vi "Example_Path to VCluster.vi"() -> ()   [LabVIEW 2015]
uses:
  <vilib>/addons/_JKI.lib/Serialization/JSON/JKI JSON Serialization.lvlib
panel:
  out "data":cluster{i32[][]}
  in  "input string":string="{\n\"History\": {\n    \"ZenParamsSpecVersion\": \"1.0.0\",\n    \"ModificationHistory\": [\n      {\n        \"DateModified\": \"19-07-2017\",\n        \"ModifiedBy\": \"SR\",\n        \"ModificationNotes\": \"FCI First version\",\n        \"DocumentVefrsion\": \"1.0.0\"\n      }\n    ],\n    \"ServiceHistory\": [\n      {\n        \"DateServiced\": \"23-03-2017\",\n        \"ServicedBy\": \"ABC\",\n        \"NextServiceDate\": \"23-03-2018\",\n        \"ServiceList\": {\n          \"CameraCalibrationDate\": \"2\",\n          \"CameraCalibrationFilePath\": \"C:\\\\Cam\",\n          \"SensorCalibration\": true,\n          \"SensorCalibNotes\": \"ReplacementDone\",\n          \"MotorCalib\": true,\n          \"MotorCalibNotes\": \"blah\"\n        },\n        \"ServiceNotes\": \"First version\"\n      },\n      {\n        \"DateServiced\": \"23-03-2017\",\n        \"ServicedBy\": \"ABC\",\n        \"NextServiceDate\": \"23-03-2018\",\n\"ServiceList\": {\n          \"CameraCalibrationDate\": \"2\",\n          \"CameraCalibrationFilePath\": \"C:\\\\Cam\",\n          \"SensorCalibration\": true,\n          \"SensorCalibNotes\": \"ReplacementDone\",\n          \"MotorCalib\": true,\n          \"MotorCalibNotes\": \"blah\"\n        },\n        \"ServiceNotes\": \"First version\"\n      }\n    ]\n  },\n  \"SystemParameters\": {\n    \"SystemName\": \"MolexGP2_001\",\n    \"SystemID\": \"GTRON1\",\n    \"CusftomerName\": \"Molex\",\n    \"Location\": \"Gandhinagar\",\n    \"InstallationfDate\": \"01-08-2015\",\n    \"NextServiceDate\": \"01-05-2017\",\n    \"CompatibleZenGageVersion\": \"2.0\",\n    \"NumberOfRacks\": 1,\n    \"TotalNumberOfCameras\": 3,\n    \"SoftwareFeatures\": {\n      \"ArduinoDiagnosticsEnableOnPowerOn\": true,\n      \"MotorDiagnosticsEnableOnPowerOn\": true,\n      \"CameraOpticsDiagnosticsEnableOnPowerOn\": false,\n      \"DefectTrackingEnable\": true,\n      \"AnalyticsEnable\": true,\n      \"DataLoggingEnable\": false,\n      \"ReportEnable\": false,\n      \"DeveloperMode\": false,\n      \"PauseOnReelCountFinish\": true,\n      \"PauseOnTotalCountFinish\": true,\n      \"DebugLevel\": 0,\n      \"SaveFailImages\": false\n    }\n  },\n  \"PartsConfigured\": [\n    {\n      \"Name\": \"102\",\n      \"NumberOfRack\": 1\n    }\n  ],\n  \"RackControllerParameters\": [\n    {\n      \"RackId\": 0,\n      \"PartsList\": [\n        {\n          \"Name\": \"102\",\n          \"ControlLimitsViolationThreshold\": {\n            \"M1\": 1,\n            \"N1\": 1\n          },\n          \"SpecificationLimitViolationThreshold\": {\n            \"M2\": 1,\n            \"N2\": 1\n          },\n          \"RejectPositionCount\": 106,\n          \"NumberOfCameras\": 1\n        },\n        {\n          \"Name\": \"122\",\n          \"ControlLimitsViolationThreshold\": {\n            \"M1\": 1,\n            \"N1\": 1\n          },\n          \"SpecificationLimitViolationThreshold\": {\n            \"M2\": 1,\n            \"N2\": 1\n          },\n          \"RejectPositionCount\": 77,\n          \"NumberOfCameras\": 3\n        },\n        {\n          \"Name\": \"145\",\n          \"ControlLimitsViolationThreshold\": {\n            \"M1\": 1,\n            \"N1\": 1\n          },\n          \"SpecificationLimitViolationThreshold\": {\n            \"M2\": 1,\n            \"N2\": 1\n          },\n          \"RejectPositionCount\": 78,\n          \"NumberOfCameras\": 3\n        },\n        {\n          \"Name\": \"162\",\n          \"ControlLimitsViolationThreshold\": {\n            \"M1\": 1,\n            \"N1\": 1\n          },\n          \"SpecificationLimitViolationThreshold\": {\n            \"M2\": 1,\n            \"N2\": 1\n          },\n          \"RejectPositionCount\": 78,\n          \"NumberOfCameras\": 3\n        },\n        {\n          \"Name\": \"182\",\n          \"ControlLimitsViolationThreshold\": {\n            \"M1\": 1,\n            \"N1\": 1\n          },\n          \"SpecificationLimitViolationThreshold\": {\n            \"M2\": 1,\n            \"N2\": 1\n          },\n          \"RejectPositionCount\": 78,\n          \"NumberOfCameras\": 3\n        },\n        {\n          \"Name\": \"175\",\n          \"ControlLimitsViolationThreshold\": {\n            \"M1\": 1,\n            \"N1\": 1\n          },\n          \"SpecificationLimitViolationThreshold\": {\n            \"M2\": 1,\n            \"N2\": 1\n          },\n          \"RejectPositionCount\": 78,\n          \"NumberOfCameras\": 3\n        },\n        {\n          \"Name\": \"130\",\n          \"ControlLimitsViolationThreshold\": {\n            \"M1\": 1,\n            \"N1\": 1\n          },\n          \"SpecificationLimitViolationThreshold\": {\n            \"M2\": 1,\n            \"N2\": 1\n          },\n          \"RejectPositionCount\": 78,\n          \"NumberOfCameras\": 3\n        },\n        {\n          \"Name\": \"142\",\n          \"ControlLimitsViolationThreshold\": {\n            \"M1\": 10,\n            \"N1\": 10\n          },\n          \"SpecificationLimitViolationThreshold\": {\n            \"M2\": 10,\n            \"N2\": 10\n          },\n          \"RejectPositionCount\": 78,\n          \"NumberOfCameras\": 3\n        },\n        {\n          \"Name\": \"160\",\n          \"ControlLimitsViolationThreshold\": {\n            \"M1\": 1,\n            \"N1\": 1\n          },\n          \"SpecificationLimitViolationThreshold\": {\n            \"M2\": 1,\n            \"N2\": 1\n          },\n          \"RejectPositionCount\": 78,\n          \"NumberOfCameras\": 3\n        }\n      ]\n    }\n  ],\n  \"CameraControllerParameters\": [\n    {\n      \"ID\": 0,\n      \"NoOfCameras\": 3,\n      \"CameraID\": [\n        0,\n        1,\n        2\n      ],\n      \"NoOfReceivers\": 1,\n      \"Diagnostics\": {\n        \"Path\": \"xxxxxx\",\n        \"LightCameraSequence\": [\n          {\n            \"Name\": \"LightCameraSequence1\",\n            \"CameraID\": 0,\n            \"LightID\": 1\n          },\n          {\n            \"Name\": \"LightCameraSequence2\",\n            \"CameraID\": 1,\n            \"LightID\": 2\n          },\n          {\n            \"Name\": \"LightCameraSequence3\",\n            \"CameraID\": 2,\n            \"LightID\": 3\n          }\n        ],\n        \"Delaytime\": 2000,\n        \"DecisionParameters\": {\n          \"Range\": [\n            70,\n            170\n          ],\n          \"AcceptancePercentage\": [\n            1,\n            20\n          ],\n          \"Comparison\": [\n            \"LesserThan\",\n            \"LesserThan\"\n          ],\n          \"AcceptableBlackBinValue\": 10000\n        },\n        \"DiagnosticsReceiverSequence\": {\n          \"ReceiverName\": \"RackController\",\n          \"ReceiverID\": 0\n        }\n      },\n      \"PartsList\": [\n        {\n          \"Name\": \"1891\",\n          \"CameraIDs\": [\n            0,\n            1\n          ],\n          \"ReceiverSequence\": [\n            {\n              \"ReceiverName\": \"Algorithm\",\n              \"ReceiverID\": 0,\n              \"NoOfActiveCameras\": 2\n            }\n          ]\n        },\n        {\n          \"Name\": \"1721\",\n          \"CameraIDs\": [\n            0,\n            1\n          ],\n          \"ReceiverSequence\": [\n            {\n              \"ReceiverName\": \"Algorithm\",\n              \"ReceiverID\": 0,\n              \"NoOfActiveCameras\": 2\n            }\n          ]\n        },\n        {\n          \"Name\": \"102\",\n          \"CameraIDs\": [\n            0\n          ],\n          \"ReceiverSequence\": [\n            {\n              \"ReceiverName\": \"RackController\",\n              \"ReceiverID\": 0,\n              \"NoOfActiveCameras\": 1\n            }\n          ]\n        },\n        {\n          \"Name\": \"122\",\n          \"CameraIDs\": [\n            0,\n            1,\n            2\n          ],\n          \"ReceiverSequence\": [\n            {\n              \"ReceiverName\": \"RackController\",\n              \"ReceiverID\": 0,\n              \"NoOfActiveCameras\": 3\n            }\n          ]\n        },\n        {\n          \"Name\": \"145\",\n          \"CameraIDs\": [\n            0,\n            1,\n            2\n          ],\n          \"ReceiverSequence\": [\n            {\n              \"ReceiverName\": \"RackController\",\n              \"ReceiverID\": 0,\n              \"NoOfActiveCameras\": 3\n            }\n          ]\n        },\n        {\n          \"Name\": \"162\",\n          \"CameraIDs\": [\n            0,\n            1,\n            2\n          ],\n          \"ReceiverSequence\": [\n            {\n              \"ReceiverName\": \"RackController\",\n              \"ReceiverID\": 0,\n              \"NoOfActiveCameras\": 3\n            }\n          ]\n        },\n        {\n          \"Name\": \"182\",\n          \"CameraIDs\": [\n            0,\n            1,\n            2\n          ],\n          \"ReceiverSequence\": [\n            {\n              \"ReceiverName\": \"RackController\",\n              \"ReceiverID\": 0,\n              \"NoOfActiveCameras\": 3\n            }\n          ]\n        },\n        {\n          \"Name\": \"175\",\n          \"CameraIDs\": [\n            0,\n            1,\n            2\n          ],\n          \"ReceiverSequence\": [\n            {\n              \"ReceiverName\": \"RackController\",\n              \"ReceiverID\": 0,\n              \"NoOfActiveCameras\": 3\n            }\n          ]\n        },\n        {\n          \"Name\": \"130\",\n          \"CameraIDs\": [\n            0,\n            1,\n            2\n          ],\n          \"ReceiverSequence\": [\n            {\n              \"ReceiverName\": \"RackController\",\n              \"ReceiverID\": 0,\n              \"NoOfActiveCameras\": 3\n            }\n          ]\n        },\n        {\n          \"Name\": \"142\",\n          \"CameraIDs\": [\n            0,\n            1,\n            2\n          ],\n          \"ReceiverSequence\": [\n            {\n              \"ReceiverName\": \"RackController\",\n              \"ReceiverID\": 0,\n              \"NoOfActiveCameras\": 3\n            }\n          ]\n        },\n        {\n          \"Name\": \"160\",\n          \"CameraIDs\": [\n            0,\n            1,\n            2\n          ],\n          \"ReceiverSequence\": [\n            {\n              \"ReceiverName\": \"RackController\",\n              \"ReceiverID\": 0,\n              \"NoOfActiveCameras\": 3\n            }\n          ]\n        }\n      ]\n    }\n  ],\n  \"ImageAcquisitionParameters\": [\n    {\n      \"Id\": 0,\n      \"SessionID\": \"Top Left\",\n      \"Type\": \"Top Left\",\n      \"Model\": \"Point grey CM3-U3-50S5m\",\n      \"InterfaceType\": \"USB3\",\n      \"SerialNumber\": \"x\",\n      \"Timeout\": 500,\n      \"GeneralCameraConfig\": [\n        {\n          \"ActiveAttribute\": \"TriggerMode\",\n          \"Value\": \"On\"\n        },\n        {\n          \"ActiveAttribute\": \"ExposureAuto\",\n          \"Value\": \"Off\"\n        },\n        {\n          \"ActiveAttribute\": \"ExposureTime\",\n          \"Value\": \"60\"\n        },\n        {\n          \"ActiveAttribute\": \"GainAuto\",\n          \"Value\": \"Off\"\n        },\n        {\n          \"ActiveAttribute\": \"Gain\",\n          \"Value\": \"0\"\n        }\n      ],\n      \"DefaultAOI\": [\n        1944,\n        1862,\n        474,\n        30\n      ],\n      \"DefaultReceiverSequence\": [\n        {\n          \"ReceiverID\": 0,\n          \"Index\": 0\n        }\n      ],\n      \"DefaultfileName\": \"ZenCAM\\\\Diagnostics\\\\Testimages\\\\top\",\n      \"Continuous\": 1,\n      \"NumberOfBuffers\": 150,\n      \"BufferNumberMode\": 0,\n      \"acquisitionTimeout\": 100,\n      \"ImageType\": 0,\n      \"Offline\": true,\n      \"ColorCameraParam\": {\n        \"PixelFormat\": \"BGRA 8 Packed\",\n        \"GammaEnable\": true,\n        \"GammaSelector\": \"sRGB\",\n        \"BalanceRationSelector\": [\n          \"Red\",\n          \"Blue\",\n          \"Green\"\n        ],\n        \"BalanceRationRaw\": [\n          95,\n          105,\n          115\n        ],\n        \"BalanceWhiteAuto\": \"Off\",\n        \"LightSourceSelector\": \"Daylight 5000 Kelvin\"\n      },\n      \"PartsList\": [\n        {\n          \"Name\": \"1891\",\n          \"ReceiverSequence\": [\n            {\n              \"ReceiverID\": 0,\n              \"Index\": 0\n            }\n          ],\n          \"AOI\": [\n            965,\n            650,\n            225,\n            250\n          ],\n          \"filePath\": \"ZenCam\\\\Test Images\\\\1891\\\\Rack1Top\"\n        },\n        {\n          \"Name\": \"1721\",\n          \"ReceiverSequence\": [\n            {\n              \"ReceiverID\": 0,\n              \"Index\": 0\n            }\n          ],\n          \"AOI\": [\n            1220,\n            670,\n            195,\n            200\n          ],\n          \"filePath\": \"ZenCam\\\\Test Images\\\\1721\\\\Rack1Top\"\n        },\n        {\n          \"Name\": \"102\",\n          \"ReceiverSequence\": [\n            {\n              \"ReceiverID\": 0,\n              \"Index\": 0\n            }\n          ],\n          \"AOI\": [\n            1600,\n            850,\n            300,\n            450\n          ],\n          \"filePath\": \"ZenCam\\\\Test Images\\\\102\\\\Top Left\"\n        },\n        {\n          \"Name\": \"122\",\n          \"ReceiverSequence\": [\n            {\n              \"ReceiverID\": 0,\n              \"Index\": 0\n            }\n          ],\n          \"AOI\": [\n            336,\n            1100,\n            1300,\n            278\n          ],\n          \"filePath\": \"ZenCam\\\\Test Images\\\\122\\\\Top Left\"\n        },\n        {\n          \"Name\": \"145\",\n          \"ReceiverSequence\": [\n            {\n              \"ReceiverID\": 0,\n              \"Index\": 0\n            }\n          ],\n          \"AOI\": [\n            480,\n            900,\n            1600,\n            500\n          ],\n          \"filePath\": \"ZenCam\\\\Test Images\\\\145\\\\Top Left\"\n        },\n        {\n          \"Name\": \"162\",\n          \"ReceiverSequence\": [\n            {\n              \"ReceiverID\": 0,\n              \"Index\": 0\n            }\n          ],\n          \"AOI\": [\n            400,\n            800,\n            1730,\n            440\n          ],\n          \"filePath\": \"ZenCam\\\\Test Images\\\\162\\\\Top Left\"\n        },\n        {\n          \"Name\": \"182\",\n          \"ReceiverSequence\": [\n            {\n              \"ReceiverID\": 0,\n              \"Index\": 0\n            }\n          ],\n          \"AOI\": [\n            464,\n            700,\n            1920,\n            600\n          ],\n          \"filePath\": \"ZenCam\\\\Test Images\\\\182\\\\Top Left\"\n        },\n        {\n          \"Name\": \"175\",\n          \"ReceiverSequence\": [\n            {\n              \"ReceiverID\": 0,\n              \"Index\": 0\n            }\n          ],\n          \"AOI\": [\n            448,\n            600,\n            2000,\n            850\n          ],\n          \"filePath\": \"ZenCam\\\\Test Images\\\\175\\\\Top Left\"\n        },\n        {\n          \"Name\": \"130\",\n          \"ReceiverSequence\": [\n            {\n              \"ReceiverID\": 0,\n              \"Index\": 0\n            }\n          ],\n          \"AOI\": [\n            400,\n            1000,\n            1420,\n            440\n          ],\n          \"filePath\": \"ZenCam\\\\Test Images\\\\130\\\\Top Left\"\n        },\n        {\n          \"Name\": \"142\",\n          \"ReceiverSequence\": [\n            {\n              \"ReceiverID\": 0,\n              \"Index\": 0\n            }\n          ],\n          \"AOI\": [\n            368,\n            930,\n            1550,\n            420\n          ],\n          \"filePath\": \"ZenCam\\\\Test Images\\\\142\\\\Top Left\"\n        },\n        {\n          \"Name\": \"160\",\n          \"ReceiverSequence\": [\n            {\n              \"ReceiverID\": 0,\n              \"Index\": 0\n            }\n          ],\n          \"AOI\": [\n            352,\n            940,\n            1800,\n            550\n          ],\n          \"filePath\": \"ZenCam\\\\Test Images\\\\160\\\\Top Left\"\n        }\n      ]\n    }\n  ],\n  \"AlgoParameters\": {\n    \"PartsList\": [\n      {\n        \"Name\": \"102\",\n        \"ImageStreams\": [\n          {\n            \"ThreadName\": \"TopRack\",\n            \"RackEnable\": true,\n            \"ThreadId\": 1,\n            \"RackId\": 1,\n            \"DifferenceParameter\": 1,\n            \"SplitCameraIDs\": [\n              0\n            ],\n            \"ImagingViews\": [\n              {\n                \"ViewName\": \"Top Left\",\n                \"ViewEnable\": true,\n                \"ImageID\": 1,\n                \"CameraID\": 0,\n                \"CalibrationFilePath\": \"Algorithm\\\\Calibration\\\\TL Calibrated Image\",\n                \"CalibImageFormat\": \"png\",\n                \"ReferenceCoordSystem\": {\n                  \"Method\": {\n                    \"Algo\": \"FCI Blob Circle\",\n                    \"BaseReference\": {\n                      \"OriginX\": 618,\n                      \"OriginY\": 464,\n                      \"Angle\": 178.38,\n                      \"AxisReference\": 0\n                    }\n                  },\n                  \"ROI\": [\n                    {\n                      \"ROI\": {\n                        \"Left\": 0,\n                        \"Top\": 260,\n                        \"Right\": 0,\n                        \"Bottom\": 700,\n                        \"Rotation\": 0\n                      },\n                      \"EdgeOptions\": {\n                        \"EdgePolarity\": 2,\n                        \"KernelSize\": 7,\n                        \"Width\": 5,\n                        \"MinimumEdgeStrength\": 50,\n                        \"InterpolationType\": 0,\n                        \"DataProcessingMethod\": 0\n                      },\n                      \"LineOptions\": {\n                        \"NumberofLines\": 1,\n                        \"Type\": 1,\n                        \"MinScore\": 10,\n                        \"MaxScore\": 1000,\n                        \"Orientation\": 0,\n                        \"AngleRange\": 30,\n                        \"AngleTolerance\": 10,\n                        \"StepSize\": 15,\n                        \"MinSNR\": 10,\n                        \"MinPoints\": 25,\n                        \"HoughIterations\": 5\n                      },\n                      \"Process\": 0,\n                      \"StepSize\": 10,\n                      \"SearchDirection\": 1,\n                      \"CircleEdgeOptions\": {\n                        \"SearchDirection\": 0,\n                        \"EdgeOptions\": {\n                          \"EdgePolarity\": 0,\n                          \"KernelSize\": 7,\n                          \"Width\": 5,\n                          \"MinimumEdgeStrength\": 50,\n                          \"InterpolationType\": 0,\n                          \"DataProcessingMethod\": 0\n                        }\n                      },\n                      \"CircleFitOptions\": {\n                        \"Process\": 3,\n                        \"StepSize\": 3,\n                        \"MAxPixelRadius\": 3\n                      },\n                      \"CircleSearchDirection\": 1,\n                      \"CurveParameters\": {\n                        \"ExtractionMode\": 0,\n                        \"EdgeThreshold\": 50,\n                        \"EdgeFilterSize\": 0,\n                        \"MinLength\": 25,\n                        \"RowSearchStepSize\": 15,\n                        \"ColSearchStepSize\": 15,\n                        \"MaxEndpointGap\": 10,\n                        \"Closed\": true,\n                        \"Subpixel\": true\n                      },\n                      \"MinimumMatchScore\": 800,\n                      \"CircleDescriptor\": {\n                        \"MinRadius\": 3,\n                        \"MaxRadius\": 200\n                      },\n                      \"EllipseDescriptor\": {\n                        \"MinMajorRadius\": 3,\n                        \"MaxMajorRadius\": 200,\n                        \"MinMinorRadius\": 3,\n                        \"MaxMinorRadius\": 100\n                      },\n                      \"ParallelLines\": {\n                        \"First\": 40,\n                        \"Second\": 55,\n                        \"Third\": 70\n                      }\n                    }\n                  ],\n                  \"Name\": \"FirstReference\",\n                  \"OverlayOptions\": {\n                    \"OverlayEnable\": false,\n                    \"OverlayText\": \"Height\",\n                    \"OverlayCoords\": [\n                      5,\n                      8\n                    ],\n                    \"OverlayAngle\": 56,\n                    \"OverlayTextSize\": 6,\n                    \"OverlayTextColor\": \"Blue\",\n                    \"OverlayROI\": true,\n                    \"OverlayRakeLine\": false,\n                    \"OverlayPoints\": false\n                  }\n                }\n              }\n            ]\n          }\n        ],\n        \"Measurements\": [\n          {\n            \"RackID\": 0,\n            \"ImageID\": 0,\n            \"CameraID\": 0,\n            \"MeasurementId\": 0,\n            \"Name\": \"EON Presence\",\n            \"AlgoName\": \"EON Presence 102\",\n            \"Type\": \"Max\",\n            \"MeasurementEnable\": true,\n            \"AlgorithmSequence\": {\n              \"RefernceEdge\": {\n                \"Enable\": true,\n                \"Method\": \"LineFinding\",\n                \"RefROI\": {\n                  \"Left\": 433,\n                  \"Top\": 292,\n                  \"Right\": 703,\n                  \"Bottom\": 665,\n                  \"Rotation\": 0\n                },\n                \"EdgeOptions\": {\n                  \"EdgePoarity\": 2,\n                  \"KernelSize\": 3,\n                  \"Width\": 3,\n                  \"MinimumEdgeStrength\": 50,\n                  \"InterpolationType\": 0,\n                  \"DataProcessingMethod\": 0\n                },\n                \"LineOptions\": {\n                  \"NumberofLines\": 1,\n                  \"Type\": 1,\n                  \"MinScore\": 10,\n                  \"MaxScore\": 1000,\n                  \"Orientation\": 0,\n                  \"AngleRange\": 10,\n                  \"AngleTolerance\": 1,\n                  \"StepSize\": 10,\n                  \"MinSNR\": 0,\n                  \"MinPoints\": 25,\n                  \"HoughIterations\": 5\n                },\n                \"SearchDirection\": 2\n              },\n              \"Measurement\": {\n                \"ROI1\": {\n                  \"Enable\": true,\n                  \"ROI\": {\n                    \"Left\": 0,\n                    \"Top\": 230,\n                    \"Right\": 0,\n                    \"Bottom\": 700,\n                    \"Rotation\": 0\n                  },\n                  \"EdgeOptions\": {\n                    \"EdgePoarity\": 0,\n                    \"KernelSize\": 3,\n                    \"Width\": 3,\n                    \"MinimumEdgeStrength\": 50,\n                    \"InterpolationType\": 0,\n                    \"DataProcessingMethod\": 0\n                  },\n                  \"LineOptions\": {\n                    \"NumberofLines\": 1,\n                    \"Type\": 1,\n                    \"MinScore\": 10,\n                    \"MaxScore\": 1000,\n                    \"Orientation\": 0,\n                    \"AngleRange\": 30,\n                    \"AngleTolerance\": 1,\n                    \"StepSize\": 3,\n                    \"MinSNR\": 0,\n                    \"MinPoints\": 25,\n                    \"HoughIterations\": 5\n                  },\n                  \"Process\": 1,\n                  \"StepSize\": 10,\n                  \"SearchDirection\": 0,\n                  \"CircleEdgeOptions\": {\n                    \"SearchDirection\": 0,\n                    \"EdgeOptions\": {\n                      \"EdgePoarity\": 2,\n                      \"KernelSize\": 3,\n                      \"Width\": 3,\n                      \"MinimumEdgeStrength\": 50,\n                      \"InterpolationType\": 1,\n                      \"DataProcessingMethod\": 1\n                    }\n                  },\n                  \"CircleFitOptions\": {\n                    \"Process\": 3,\n                    \"StepSize\": 3,\n                    \"MAxPixelRadius\": 3.85\n                  },\n                  \"CircleSearchDirection\": 1,\n                  \"CurveParameters\": {\n                    \"ExtractionMode\": 0,\n                    \"EdgeThreshold\": 50,\n                    \"EdgeFilterSize\": 0,\n                    \"MinLength\": 25,\n                    \"RowSearchStepSize\": 15,\n                    \"ColSearchStepSize\": 15,\n                    \"MaxEndpointGap\": 10,\n                    \"Closed\": true,\n                    \"Subpixel\": true\n                  },\n                  \"MinimumMatchScore\": 800,\n                  \"CircleDescriptor\": {\n                    \"MinRadius\": 3,\n                    \"MaxRadius\": 200\n                  },\n                  \"EllipseDescriptor\": {\n                    \"MinMajorRadius\": 2,\n                    \"MaxMajorRadius\": 200,\n                    \"MinMinorRadius\": 2,\n                    \"MaxMinorRadius\": 100\n                  }\n                },\n                \"ROI2\": {\n                  \"Enable\": true,\n                  \"ROI\": {\n                    \"Left\": 143,\n                    \"Top\": 244,\n                    \"Right\": 217,\n                    \"Bottom\": 456,\n                    \"Rotation\": 0.01\n                  },\n                  \"EdgeOptions\": {\n                    \"EdgePoarity\": 0,\n                    \"KernelSize\": 3,\n                    \"Width\": 3,\n                    \"MinimumEdgeStrength\": 50,\n                    \"InterpolationType\": 0,\n                    \"DataProcessingMethod\": 0\n                  },\n                  \"LineOptions\": {\n                    \"NumberofLines\": 1,\n                    \"Type\": 1,\n                    \"MinScore\": 10,\n                    \"MaxScore\": 1000,\n                    \"Orientation\": 0,\n                    \"AngleRange\": 30,\n                    \"AngleTolerance\": 1,\n                    \"StepSize\": 3,\n                    \"MinSNR\": 0,\n                    \"MinPoints\": 25,\n                    \"HoughIterations\": 5\n                  },\n                  \"Process\": 1,\n                  \"StepSize\": 10,\n                  \"SearchDirection\": 2,\n                  \"CircleEdgeOptions\": {\n                    \"SearchDirection\": 0,\n                    \"EdgeOptions\": {\n                      \"EdgePoarity\": 2,\n                      \"KernelSize\": 3,\n                      \"Width\": 3,\n                      \"MinimumEdgeStrength\": 50,\n                      \"InterpolationType\": 1,\n                      \"DataProcessingMethod\": 1\n                    }\n                  },\n                  \"CircleFitOptions\": {\n                    \"Process\": 3,\n                    \"StepSize\": 3,\n                    \"MAxPixelRadius\": 3.85\n                  },\n                  \"CircleSearchDirection\": 1,\n                  \"CurveParameters\": {\n                    \"ExtractionMode\": 0,\n                    \"EdgeThreshold\": 50,\n                    \"EdgeFilterSize\": 0,\n                    \"MinLength\": 25,\n                    \"RowSearchStepSize\": 15,\n                    \"ColSearchStepSize\": 15,\n                    \"MaxEndpointGap\": 10,\n                    \"Closed\": true,\n                    \"Subpixel\": true\n                  },\n                  \"MinimumMatchScore\": 800,\n                  \"CircleDescriptor\": {\n                    \"MinRadius\": 3,\n                    \"MaxRadius\": 200\n                  },\n                  \"EllipseDescriptor\": {\n                    \"MinMajorRadius\": 2,\n                    \"MaxMajorRadius\": 200,\n                    \"MinMinorRadius\": 2,\n                    \"MaxMinorRadius\": 100\n                  }\n                }\n              }\n            },\n            \"MathExpression\": {\n              \"Algorithm\": \"Default\",\n              \"MathExpression\": \"a = 1*a + 0\",\n              \"ResultVariable\": \"a\"\n            },\n            \"ResultVariableCluster\": {\n              \"RVName\": \"a\",\n              \"RVSequence\": \"MeasROI1\",\n              \"RVIndex\": 1,\n              \"RVID\": 1,\n              \"RVValue\": 22.6\n            },\n            \"CalibrationCoefficients\": {\n              \"A1\": 1,\n              \"A2\": 0,\n              \"A3\": 0\n            },\n            \"UserCalibCoefficients\": {\n              \"UserCorrectionLinearityCoeff\": 1,\n              \"UserCorrectionBiasCoeff\": 0\n            },\n            \"SpecValues\": {\n              \"LCL\": 1500,\n              \"UCL\": 2500,\n              \"LSL\": 1500,\n              \"USL\": 2500,\n              \"NominalValue\": 2000\n            },\n            \"OverlayOptions\": {\n              \"OverlayEnable\": false,\n              \"OverlayText\": \"Width\",\n              \"OverlayCoords\": [\n                5,\n                8\n              ],\n              \"OverlayAngle\": 56,\n              \"OverlayTextSize\": 6,\n              \"OverlayTextColor\": \"Blue\",\n              \"OverlayROI\": false,\n              \"OverlayRakeLine\": false,\n              \"OverlayPoints\": false\n            },\n            \"DatalogEnable\": true,\n            \"DisplayIcon\": \"C:\\\\Desktop\\\\displayimage.png\"\n          }\n        ]\n      }\n    ],\n    \"AlgoDefaultParameters\": {\n      \"AlgoName\": \"MaxClamp\",\n      \"Enable\": true,\n      \"AlgorithmSequenceDefault\": {\n        \"RefernceEdgeDefault\": {\n          \"Method\": \"LineFinding\",\n          \"RefROI\": {\n            \"Left\": 1014,\n            \"Top\": 95,\n            \"Right\": 1290,\n            \"Bottom\": 520,\n            \"Rotation\": 0\n          },\n          \"EdgeOptions\": {\n            \"EdgePoarity\": 0,\n            \"KernelSize\": 3,\n            \"Width\": 3,\n            \"MinimumEdgeStrength\": 50,\n            \"InterpolationType\": 1,\n            \"DataProcessingMethod\": 1\n          },\n          \"LineOptions\": {\n            \"NumberofLines\": 1,\n            \"Type\": 1,\n            \"MinScore\": 10,\n            \"MaxScore\": 1000,\n            \"Orientation\": 0,\n            \"AngleRange\": 10,\n            \"AngleTolerance\": 1,\n            \"StepSize\": 3,\n            \"MinSNR\": 0,\n            \"MinPoints\": 25,\n            \"HoughIterations\": 5\n          },\n          \"SearchDirection\": 2\n        },\n        \"MeasurementDefault\": {\n          \"ROI1\": {\n            \"ROI\": {\n              \"Left\": 100,\n              \"Top\": 150,\n              \"Right\": 400,\n              \"Bottom\": 700,\n              \"Rotation\": 0\n            },\n            \"EdgeOptions\": {\n              \"EdgePoarity\": 0,\n              \"KernelSize\": 3,\n              \"Width\": 3,\n              \"MinimumEdgeStrength\": 50,\n              \"InterpolationType\": 1,\n              \"DataProcessingMethod\": 1\n            },\n            \"LineOptions\": {\n              \"NumberofLines\": 1,\n              \"Type\": 1,\n              \"MinScore\": 10,\n              \"MaxScore\": 1000,\n              \"Orientation\": 0,\n              \"AngleRange\": 10,\n              \"AngleTolerance\": 1,\n              \"StepSize\": 3,\n              \"MinSNR\": 0,\n              \"MinPoints\": 25,\n              \"HoughIterations\": 5\n            },\n            \"Process\": 1,\n            \"StepSize\": 10,\n            \"SearchDirection\": 0,\n            \"CircleEdgeOptions\": {\n              \"SearchDirection\": 1,\n              \"EdgeOptions\": {\n                \"EdgePoarity\": 0,\n                \"KernelSize\": 3,\n                \"Width\": 3,\n                \"MinimumEdgeStrength\": 50,\n                \"InterpolationType\": 1,\n                \"DataProcessingMethod\": 1\n              }\n            },\n            \"CircleFitOptions\": {\n              \"Process\": 3,\n              \"StepSize\": 3,\n              \"MAxPixelRadius\": 3\n            },\n            \"CircleSearchDirection\": 1,\n            \"CurveParameters\": {\n              \"ExtractionMode\": 0,\n              \"EdgeThreshold\": 50,\n              \"EdgeFilterSize\": 0,\n              \"MinLength\": 25,\n              \"RowSearchStepSize\": 15,\n              \"ColSearchStepSize\": 15,\n              \"MaxEndpointGap\": 10,\n              \"Closed\": 0,\n              \"Subpixel\": 0\n            },\n            \"MinimumMatchScore\": 800,\n            \"CircleDescriptor\": {\n              \"MinRadius\": 3,\n              \"MaxRadius\": 200\n            },\n            \"EllipseDescriptor\": {\n              \"MinMajorRadius\": 2,\n              \"MaxMajorRadius\": 200,\n              \"MinMinorRadius\": 2,\n              \"MaxMinorRadius\": 100\n            },\n            \"OverlayOptions\": {\n              \"OverlayEnable\": true,\n              \"OverlayText\": \"Collar Width\",\n              \"OverlayCoords\": [\n                5,\n                8\n              ],\n              \"OverlayAngle\": 56,\n              \"OverlayTextSize\": 6,\n              \"OverlayTextColor\": \"Red\"\n            },\n            \"ResultVariable\": \"M1\"\n          },\n          \"ROI2\": {\n            \"ROI\": {\n              \"Left\": 100,\n              \"Top\": 150,\n              \"Right\": 400,\n              \"Bottom\": 700,\n              \"Rotation\": 0\n            },\n            \"EdgeOptions\": {\n              \"EdgePoarity\": 0,\n              \"KernelSize\": 3,\n              \"Width\": 3,\n              \"MinimumEdgeStrength\": 50,\n              \"InterpolationType\": 1,\n              \"DataProcessingMethod\": 1\n            },\n            \"LineOptions\": {\n              \"NumberofLines\": 1,\n              \"Type\": 1,\n              \"MinScore\": 10,\n              \"MaxScore\": 1000,\n              \"Orientation\": 0,\n              \"AngleRange\": 10,\n              \"AngleTolerance\": 1,\n              \"StepSize\": 3,\n              \"MinSNR\": 0,\n              \"MinPoints\": 25,\n              \"HoughIterations\": 5\n            },\n            \"Process\": 1,\n            \"StepSize\": 10,\n            \"SearchDirection\": 0,\n            \"CircleEdgeOptions\": {\n              \"SearchDirection\": 1,\n              \"EdgeOptions\": {\n                \"EdgePoarity\": 0,\n                \"KernelSize\": 3,\n                \"Width\": 3,\n                \"MinimumEdgeStrength\": 50,\n                \"InterpolationType\": 1,\n                \"DataProcessingMethod\": 1\n              }\n            },\n            \"CircleFitOptions\": {\n              \"Process\": 3,\n              \"StepSize\": 3,\n              \"MaxPixelRadius\": 3\n            },\n            \"CircleSearchDirection\": 1,\n            \"CurveParameters\": {\n              \"ExtractionMode\": 0,\n              \"EdgeThreshold\": 50,\n              \"EdgeFilterSize\": 0,\n              \"MinLength\": 25,\n              \"RowSearchStepSize\": 15,\n              \"ColSearchStepSize\": 15,\n              \"MaxEndpointGap\": 10,\n              \"Closed\": 0,\n              \"Subpixel\": 0\n            },\n            \"MinimumMatchScore\": 800,\n            \"CircleDescriptor\": {\n              \"MinRadius\": 3,\n              \"MaxRadius\": 200\n            },\n            \"EllipseDescriptor\": {\n              \"MinMajorRadius\": 2,\n              \"MaxMajorRadius\": 200,\n              \"MinMinorRadius\": 2,\n              \"MaxMinorRadius\": 100\n            },\n            \"OverlayOptions\": {\n              \"OverlayEnable\": true,\n              \"OverlayText\": \"Collar Width\",\n              \"OverlayCoords\": [\n                5,\n                8\n              ],\n              \"OverlayAngle\": 56,\n              \"OverlayTextSize\": 6,\n              \"OverlayTextColor\": \"Red\"\n            },\n            \"ResultVariable\": \"M2\"\n          }\n        },\n        \"MathExpressionDefault\": {\n          \"Algorithm\": \"Math1\",\n          \"MathExpression\": \"M2-M1\",\n          \"ResultVariable\": \"M3\"\n        }\n      },\n      \"CalibrationCoefficients\": {\n        \"A1\": 13,\n        \"A2\": 8.7,\n        \"A3\": 67.9\n      },\n      \"UserCalibCoefficients\": {\n        \"UserCorrectionBiasCoeff\": 56,\n        \"UserCorrectionLinearityCoeff\": 45\n      },\n      \"OverlayOptions\": {\n        \"OverlayEnable\": true,\n        \"OverlayText\": \"Collar Width\",\n        \"OverlayCoords\": [\n          5,\n          8\n        ],\n        \"OverlayAngle\": 56,\n        \"OverlayTextSize\": 6,\n        \"OverlayTextColor\": \"Red\"\n      },\n      \"DatalogEnable\": true,\n      \"DisplayIcon\": \"C:\\\\Desktop\\\\displayimage.png\"\n    }\n  },\n  \"MachineInterfaceRecipeOpcodes\": {\n    \"DeviceReadiness\": {\n      \"Ping\": [\n        \"01QRY1111\"\n      ],\n      \"PingResponse\": [\n        \"11YES11\"\n      ]\n    },\n    \"Initialization\": [\n      {\n        \"Clear\": [\n          \"01CLR1111\"\n        ]\n      },\n      {\n        \"Debug\": [\n          \"01DBG0011\"\n        ]\n      },\n      {\n        \"PinModeConfiguration\": [\n          \"01PMD39111\",\n          \"01PMD38111\",\n          \"01PMD40111\",\n          \"01PMD42111\",\n          \"01PMD16111\",\n          \"01PMD43111\",\n          \"01PMD34111\",\n          \"01PMD35111\",\n          \"01PMD36111\",\n          \"01PMD37111\",\n          \"01PMD30111\",\n          \"01PMD31111\",\n          \"01PMD32111\",\n          \"01PMD33111\",\n          \"01PMD46111\",\n          \"01PMD47111\",\n          \"01PMD48111\",\n          \"01PMD49111\",\n          \"01PMD13011\",\n          \"01PMD12011\",\n          \"01PMD11011\",\n          \"01PMD10011\",\n          \"01PMD09011\",\n          \"01PMD08011\",\n          \"01PMD02011\",\n          \"01PMD03011\",\n          \"01PMD05011\",\n          \"01PMD06011\",\n          \"01PMD04011\",\n          \"01PMD14011\",\n          \"01PMD52111\",\n          \"01PMD53111\",\n          \"01LOW3311\",\n          \"01LOW5211\",\n          \"01LOW5311\",\n          \"01HGH4211\",\n          \"01HGH1611\",\n          \"01HGH4311\",\n          \"01PMD07011\"\n        ]\n      },\n      {\n        \"EventSequenceOpcodes\": [\n          \"10ENT11341510430004100011\",\n          \"10ENT12361510410004150011\",\n          \"10ENT134211141029011\",\n          \"10ENT1439151523029011\",\n          \"10ENT15421210101011\",\n          \"10ENT161611171029011\",\n          \"10ENT1738151823029011\",\n          \"10ENT18161210101011\",\n          \"10ENT1943112101029011\",\n          \"10ENT210401521123029011\",\n          \"10ENT211431210101011\",\n          \"10ENT2124211213101511\",\n          \"10ENT213391521423025011\",\n          \"10ENT2144212215101011\",\n          \"10ENT2151611216101511\",\n          \"10ENT216381521723025011\",\n          \"10ENT2171612218101011\",\n          \"10ENT2184311219101511\",\n          \"10ENT219401522023025011\",\n          \"10ENT220431210101011\"\n        ]\n      },\n      {\n        \"LogicalOperations\": [\n          \"10LGC101010101011\"\n        ]\n      },\n      {\n        \"ConditionalOperations\": [\n          \"10CND10101011\"\n        ]\n      },\n      {\n        \"InterruptTriggerBindingOpcodes\": [\n          \"10SET2211111\",\n          \"10SET2221211\",\n          \"10SET2231311\",\n          \"10SET2241611\",\n          \"10SET2251911\",\n          \"10SET22621211\",\n          \"10SET2084100011\",\n          \"10SET2094100011\",\n          \"10SET2104100011\",\n          \"10SET2114100011\",\n          \"10SET2124100011\",\n          \"10SET2134100011\"\n        ]\n      },\n      {\n        \"PinInformation\": [\n          \"01STM4611\",\n          \"01WND4711\",\n          \"01S1U0411\",\n          \"01S1L0611\",\n          \"01S2U0511\",\n          \"01LOW3511\"\n        ]\n      }\n    ],\n    \"OpenLimitSwitchStatus\": [\n      {\n        \"LimitSwitchStatusCheck\": [\n          \"01PST0911\"\n        ],\n        \"LimitSwitchStatusResponse\": [\n          \"1109111\",\n          \"1109011\"\n        ]\n      }\n    ],\n    \"MotorDiagnostics\": [\n      {\n        \"GuideOpen\": [\n          \"01LOW3711\",\n          \"01ENL095500001111\",\n          \"10DLY55000011\",\n          \"01EVT2211\",\n          \"01LPI0911\"\n        ],\n        \"GuideOpenResponse\": [\n          \"11P0911\",\n          \"11W0911\"\n        ],\n        \"GuideClose\": [\n          \"01HGH3711\",\n          \"01ENL085500001111\",\n          \"10DLY55000011\",\n          \"01EVT2211\",\n          \"01LPI0811\"\n        ],\n        \"GuideCloseResponse\": [\n          \"11P0811\",\n          \"11W0811\"\n        ],\n        \"RotateReelerMotor\": [\n          \"10DLY4300011\",\n          \"01EVT2111\",\n          \"01LPI0011\"\n        ]\n      }\n    ],\n    \"HardwareButtonDiagnostics\": {\n      \"Run\": [\n        \"01ENL135500001111\",\n        \"01DBL1311\"\n      ],\n      \"Pause\": [\n        \"01ENL125500001111\",\n        \"01DBL1211\"\n      ],\n      \"Stop\": [\n        \"01ENL115500001111\",\n        \"01DBL1111\"\n      ],\n      \"BuzzerOff\": [\n        \"01ENL105500001111\",\n        \"01DBL1011\"\n      ]\n    },\n    \"TriggerLightCameraSequence\": [\n      {\n        \"Name\": \"LightCameraSequence1\",\n        \"On\": [\n          \"01EVT2311\"\n        ],\n        \"Off\": [\n          \"01HGH4211\"\n        ]\n      },\n      {\n        \"Name\": \"LightCameraSequence2\",\n        \"On\": [\n          \"01EVT2411\"\n        ],\n        \"Off\": [\n          \"01HGH1611\"\n        ]\n      },\n      {\n        \"Name\": \"LightCameraSequence3\",\n        \"On\": [\n          \"01EVT2511\"\n        ],\n        \"Off\": [\n          \"01HGH4311\"\n        ]\n      }\n    ],\n    \"SensorDiagnostics\": [\n      {\n        \"Name\": \"Sensor1\",\n        \"Opcodes\": [\n          \"01ENL025350001111\",\n          \"01SEN0211\",\n          \"01HGH4811\",\n          \"10SET20221211\"\n        ]\n      },\n      {\n        \"Name\": \"Sensor2\",\n        \"Opcodes\": [\n          \"01ENL035550001111\",\n          \"01SEN0311\",\n          \"01HGH4911\",\n          \"10SET20321211\"\n        ]\n      }\n    ],\n    \"TowerLampDiagnostics\": {\n      \"RedLamp\": [\n        \"01HGH3011\",\n        \"01LOW3011\"\n      ],\n      \"YellowLamp\": [\n        \"01HGH3111\",\n        \"01LOW3111\"\n      ],\n      \"GreenLamp\": [\n        \"01HGH3211\",\n        \"01LOW3211\"\n      ],\n      \"Buzzer\": [\n        \"01HGH3311\",\n        \"01LOW3311\"\n      ]\n    },\n    \"Select\": [\n      {\n        \"HardwareButtonStatus\": [\n          \"01ENL135550001111\",\n          \"01DBL1211\",\n          \"01DBL1111\",\n          \"01DBL1011\",\n          \"01DBL0811\",\n          \"01DBL0911\"\n        ]\n      },\n      {\n        \"SwitchOnYellow\": [\n          \"01HGH3111\"\n        ]\n      },\n      {\n        \"StampingWindingControl\": [\n          \"01LOW4611\",\n          \"01LOW4711\"\n        ]\n      }\n    ],\n    \"Run\": {\n      \"HardwareButtonStatus\": [\n        \"01LOW3511\",\n        \"01DBL1311\",\n        \"01ENL125500001111\",\n        \"01ENL115500001111\",\n        \"01DBL1011\",\n        \"01DBL0811\",\n        \"01DBL0911\",\n        \"01LOW4611\",\n        \"01LOW4711\"\n      ],\n      \"Pass\": {\n        \"TowerLampStatus\": [\n          \"01LOW3011\",\n          \"01LOW3111\",\n          \"01HGH3211\",\n          \"01LOW3311\"\n        ]\n      }\n    },\n    \"Pause\": {\n      \"PauseButtonPress\": [\n        {\n          \"StampingWindingControl\": [\n            \"01SMT2111\",\n            \"01HGH4611\",\n            \"01HGH4711\"\n          ]\n        },\n        {\n          \"StampingWindingControl\": [\n            \"01HGH4611\",\n            \"01HGH4711\"\n          ]\n        },\n        {\n          \"DisableSensor\": []\n        },\n        {\n          \"TowerLampStatus\": [\n            \"01LOW3011\",\n            \"01HGH3111\",\n            \"01LOW3211\",\n            \"01LOW3311\"\n          ]\n        },\n        {\n          \"HardwareButtonStatus\": [\n            \"01ENL135500001111\",\n            \"01DBL1211\",\n            \"01ENL115500001111\",\n            \"01DBL1011\",\n            \"01DBL0811\",\n            \"01DBL0911\"\n          ]\n        }\n      ],\n      \"Fail\": [\n        {\n          \"DisableSensors\": [\n            \"01SMT2111\"\n          ]\n        },\n        {\n          \"TowerLampStatus\": [\n            \"01HGH3011\",\n            \"01LOW3111\",\n            \"01LOW3211\",\n            \"01HGH3311\"\n          ]\n        },\n        {\n          \"HardwareButtonStatus\": [\n            \"01ENL135500001111\",\n            \"01DBL1211\",\n            \"01ENL115500001111\",\n            \"01ENL105500001111\",\n            \"01DBL0811\",\n            \"01DBL0911\"\n          ]\n        }\n      ],\n      \"BuzzerOffButtonPress\": [\n        \"01LOW3311\"\n      ]\n    },\n    \"Exit\": {\n      \"Shutdown\": [\n        \"01EXT1411\",\n        \"01ENL145500001111\",\n        \"01PWR5211\"\n      ]\n    },\n    \"DHBLS\": [\n      {\n        \"DisableHardwareButtons\": [\n          \"01DBL1311\",\n          \"01DBL1211\",\n          \"01DBL1111\",\n          \"01DBL1011\",\n          \"01DBL0811\",\n          \"01DBL0911\"\n        ]\n      },\n      {\n        \"TowerLampsOff\": [\n          \"01LOW3011\",\n          \"01LOW3111\",\n          \"01LOW3211\",\n          \"01LOW3311\"\n        ]\n      },\n      {\n        \"PowerOffSensors\": [\n          \"01LOW4811\",\n          \"01LOW4911\"\n        ]\n      },\n      {\n        \"DisableSensors\": [\n          \"01DBL0211\",\n          \"01DBL0311\"\n        ]\n      },\n      {\n        \"StampingWindingControl\": [\n          \"01HGH4611\",\n          \"01HGH4711\",\n          \"01SMT2111\"\n        ]\n      }\n    ],\n    \"PartsList\": [\n      {\n        \"Name\": \"102\",\n        \"RackDependentOpcodes\": [\n          {\n            \"MotorStepsForReadyToInsert\": [\n              \"01HGH3711\",\n              \"10DLY51350211\",\n              \"01EVT2211\",\n              \"01LPI0011\"\n            ],\n            \"MotorStepsForReadyToRun\": [\n              \"01HGH3711\",\n              \"10DLY4110311\",\n              \"01EVT2211\",\n              \"01LPI0011\"\n            ],\n            \"SetIndex\": [\n              \"10SET20220311\"\n            ],\n            \"EnableAndPowerOnSensor\": [\n              \"01ENL025350001111\",\n              \"01SEN0211\",\n              \"01HGH4811\",\n              \"01SST2111\"\n            ]\n          }\n        ]\n      },\n      {\n        \"Name\": \"182\",\n        \"RackDependentOpcodes\": [\n          {\n            \"MotorStepsForReadyToInsert\": [\n              \"01HGH3711\",\n              \"10DLY4367711\",\n              \"01EVT2211\",\n              \"01LPI0011\"\n            ],\n            \"MotorStepsForReadyToRun\": [\n              \"01HGH3711\",\n              \"10DLY4130311\",\n              \"01EVT2211\",\n              \"01LPI0011\"\n            ],\n            \"SetIndex\": [\n              \"10SET20221211\"\n            ],\n            \"EnableAndPowerOnSensor\": [\n              \"01ENL025350001111\",\n              \"01SEN0211\",\n              \"01HGH4811\",\n              \"01SST2111\"\n            ]\n          }\n        ]\n      },\n      {\n        \"Name\": \"145\",\n        \"RackDependentOpcodes\": [\n          {\n            \"MotorStepsForReadyToInsert\": [\n              \"01HGH3711\",\n              \"10DLY4521711\",\n              \"01EVT2211\",\n              \"01LPI0011\"\n            ],\n            \"MotorStepsForReadyToRun\": [\n              \"01HGH3711\",\n              \"10DLY4130311\",\n              \"01EVT2211\",\n              \"01LPI0011\"\n            ],\n            \"SetIndex\": [\n              \"10SET20221211\"\n            ],\n            \"EnableAndPowerOnSensor\": [\n              \"01ENL025350001111\",\n              \"01SEN0211\",\n              \"01HGH4811\",\n              \"01SST2111\"\n            ]\n          }\n        ]\n      },\n      {\n        \"Name\": \"142\",\n        \"RackDependentOpcodes\": [\n          {\n            \"MotorStepsForReadyToInsert\": [\n              \"01HGH3711\",\n              \"10DLY4890011\",\n              \"01EVT2211\",\n              \"01LPI0011\"\n            ],\n            \"MotorStepsForReadyToRun\": [\n              \"01HGH3711\",\n              \"10DLY395011\",\n              \"01EVT2211\",\n              \"01LPI0011\"\n            ],\n            \"SetIndex\": [\n              \"10SET20221211\"\n            ],\n            \"EnableAndPowerOnSensor\": [\n              \"01ENL025350001111\",\n              \"01SEN0211\",\n              \"01HGH4811\",\n              \"01SST2111\"\n            ]\n          }\n        ]\n      },\n      {\n        \"Name\": \"122\",\n        \"RackDependentOpcodes\": [\n          {\n            \"MotorStepsForReadyToInsert\": [\n              \"01HGH3711\",\n              \"10DLY51200411\",\n              \"01EVT2211\",\n              \"01LPI0011\"\n            ],\n            \"MotorStepsForReadyToRun\": [\n              \"01HGH3711\",\n              \"10DLY4110311\",\n              \"01EVT2211\",\n              \"01LPI0011\"\n            ],\n            \"SetIndex\": [\n              \"10SET20221211\"\n            ],\n            \"EnableAndPowerOnSensor\": [\n              \"01ENL025350001111\",\n              \"01SEN0211\",\n              \"01HGH4811\",\n              \"01SST2111\"\n            ]\n          }\n        ]\n      },\n      {\n        \"Name\": \"130\",\n        \"RackDependentOpcodes\": [\n          {\n            \"MotorStepsForReadyToInsert\": [\n              \"01HGH3711\",\n              \"10DLY4900011\",\n              \"01EVT2211\",\n              \"01LPI0011\"\n            ],\n            \"MotorStepsForReadyToRun\": [\n              \"01HGH3711\",\n              \"10DLY4110311\",\n              \"01EVT2211\",\n              \"01LPI0011\"\n            ],\n            \"SetIndex\": [\n              \"10SET20221211\"\n            ],\n            \"EnableAndPowerOnSensor\": [\n              \"01ENL025350001111\",\n              \"01SEN0211\",\n              \"01HGH4811\",\n              \"01SST2111\"\n            ]\n          }\n        ]\n      },\n      {\n        \"Name\": \"160\",\n        \"RackDependentOpcodes\": [\n          {\n            \"MotorStepsForReadyToInsert\": [\n              \"01HGH3711\",\n              \"10DLY4321111\",\n              \"01EVT2211\",\n              \"01LPI0011\"\n            ],\n            \"MotorStepsForReadyToRun\": [\n              \"01HGH3711\",\n              \"10DLY4110311\",\n              \"01EVT2211\",\n              \"01LPI0011\"\n            ],\n            \"SetIndex\": [\n              \"10SET20221211\"\n            ],\n            \"EnableAndPowerOnSensor\": [\n              \"01ENL025350001111\",\n              \"01SEN0211\",\n              \"01HGH4811\",\n              \"01SST2111\"\n            ]\n          }\n        ]\n      },\n      {\n        \"Name\": \"162\",\n        \"RackDependentOpcodes\": [\n          {\n            \"MotorStepsForReadyToInsert\": [\n              \"01HGH3711\",\n              \"10DLY4600011\",\n              \"01EVT2211\",\n              \"01LPI0011\"\n            ],\n            \"MotorStepsForReadyToRun\": [\n              \"01HGH3711\",\n              \"10DLY4110311\",\n              \"01EVT2211\",\n              \"01LPI0011\"\n            ],\n            \"SetIndex\": [\n              \"10SET20221211\"\n            ],\n            \"EnableAndPowerOnSensor\": [\n              \"01ENL025350001111\",\n              \"01SEN0211\",\n              \"01HGH4811\",\n              \"01SST2111\"\n            ]\n          }\n        ]\n      },\n      {\n        \"Name\": \"175\",\n        \"RackDependentOpcodes\": [\n          {\n            \"MotorStepsForReadyToInsert\": [\n              \"01HGH3711\",\n              \"10DLY1111\",\n              \"01EVT2211\",\n              \"01LPI0011\"\n            ],\n            \"MotorStepsForReadyToRun\": [\n              \"01HGH3711\",\n              \"10DLY4110311\",\n              \"01EVT2211\",\n              \"01LPI0011\"\n            ],\n            \"SetIndex\": [\n              \"10SET20221211\"\n            ],\n            \"EnableAndPowerOnSensor\": [\n              \"01ENL025350001111\",\n              \"01SEN0211\",\n              \"01HGH4811\",\n              \"01SST2111\"\n            ]\n          }\n        ]\n      }\n    ],\n    \"HardwareButtonPressed\": {\n      \"RunButtonPress\": [\n        \"11P1311\"\n      ],\n      \"PauseButtonPress\": [\n        \"11P1211\"\n      ],\n      \"StopButtonPress\": [\n        \"11P1111\"\n      ],\n      \"BuzzerOffButtonPress\": [\n        \"11P1011\"\n      ]\n    },\n    \"ReadyPositionReached\": [\n      \"11P0011\"\n    ],\n    \"IncorrectOpcode\": [\n      \"11FLS11\"\n    ]\n  },\n  \"AnalyticsParameters\": {\n    \"UpdateRateCategories\": {\n      \"LOW\": {\n        \"SampleElapsed\": 100,\n        \"TimeElapsed\": 4\n      },\n      \"MEDIUM\": {\n        \"SampleElapsed\": 20,\n        \"TimeElapsed\": 8\n      },\n      \"HIGH\": {\n        \"SampleElapsed\": 1,\n        \"TimeElapsed\": 5\n      }\n    },\n    \"AnalyticsForPartsList\": [\n      {\n        \"Name\": \"102\",\n        \"InitializationValues\": {\n          \"RowsIn2DArray\": 9000,\n          \"ColumnsIn2DArray\": 13,\n          \"SamplesToDisplay\": 100,\n          \"UpdateRate\": \"MEDIUM\"\n        },\n        \"PlotParameters\": {\n          \"Trend\": [\n            {\n              \"TrendID\": 1,\n              \"PlotEnable\": true,\n              \"PlotTitle\": \"EON Presence Summary\",\n              \"PlotCaptionFont\": {\n                \"FontName\": \"Times New Roman\",\n                \"FontSize\": 15,\n                \"IsBold\": true,\n                \"IsItalic\": false,\n                \"IsUnderline\": false,\n                \"IsStrikeout\": false,\n                \"FontColor\": \"Black\"\n              },\n              \"XLabel\": \"Frequency Count\",\n              \"XLabelFont\": {\n                \"FontName\": \"Times New Roman\",\n                \"FontSize\": 15,\n                \"IsBold\": true,\n                \"IsItalic\": false,\n                \"IsUnderline\": false,\n                \"IsStrikeout\": false,\n                \"FontColor\": \"Black\"\n              },\n              \"SamplesToDisplay\": 100,\n              \"Channels\": [\n                {\n                  \"Label\": \"EON Presence Value\",\n                  \"YLabelFont\": {\n                    \"FontName\": \"Times New Roman\",\n                    \"FontSize\": 15,\n                    \"IsBold\": true,\n                    \"IsItalic\": false,\n                    \"IsUnderline\": false,\n                    \"IsStrikeout\": false,\n                    \"FontColor\": \"Black\"\n                  },\n                  \"MeasurementID\": 1,\n                  \"PlotColor\": \"Pink\",\n                  \"PointShape\": \"circle\",\n                  \"ShowOnGraph\": true\n                }\n              ]\n            }\n          ],\n          \"Histogram\": [\n            {\n              \"HistogramID\": 1,\n              \"PlotEnable\": true,\n              \"PlotTitle\": \"EON Presence Histogram Summary\",\n              \"PlotLabelFont\": {\n                \"FontName\": \"Times New Roman\",\n                \"FontSize\": 15,\n                \"IsBold\": true,\n                \"IsItalic\": false,\n                \"IsUnderline\": false,\n                \"IsStrikeout\": false,\n                \"FontColor\": \"Black\"\n              },\n              \"XLabel\": \"Height count\",\n              \"XLabelFont\": {\n                \"FontName\": \"Calibri\",\n                \"FontSize\": 15,\n                \"IsBold\": true,\n                \"IsItalic\": false,\n                \"IsUnderline\": false,\n                \"IsStrikeout\": false,\n                \"FontColor\": \"Black\"\n              },\n              \"YLabel\": \"EON Presence Values\",\n              \"YLabelFont\": {\n                \"FontName\": \"Times New Roman\",\n                \"FontSize\": 15,\n                \"IsBold\": true,\n                \"IsItalic\": false,\n                \"IsUnderline\": false,\n                \"IsStrikeout\": false,\n                \"FontColor\": \"Black\"\n              },\n              \"MeasurementID\": 1,\n              \"PlotColor\": \"Pink\",\n              \"SamplesToDisplay\": 10\n            }\n          ],\n          \"BarPlot\": [\n            {\n              \"BarPlotID\": 1,\n              \"BarValuesID\": 0,\n              \"PlotEnable\": true,\n              \"PlotLabel\": \"Production Summary\",\n              \"PlotLabelFont\": {\n                \"FontName\": \"Times New Roman\",\n                \"FontSize\": 15,\n                \"IsBold\": true,\n                \"IsItalic\": false,\n                \"IsUnderline\": false,\n                \"IsStrikeout\": false,\n                \"FontColor\": \"Black\"\n              },\n              \"XLabel\": \" Terminal Production\",\n              \"XLabelFont\": {\n                \"FontName\": \"Times New Roman\",\n                \"FontSize\": 15,\n                \"IsBold\": true,\n                \"IsItalic\": false,\n                \"IsUnderline\": false,\n                \"IsStrikeout\": false,\n                \"FontColor\": \"Black\"\n              },\n              \"YLabel\": \"Total Production Count\",\n              \"YLabelFont\": {\n                \"FontName\": \"Times New Roman\",\n                \"FontSize\": 15,\n                \"IsBold\": true,\n                \"IsItalic\": false,\n                \"IsUnderline\": false,\n                \"IsStrikeout\": false,\n                \"FontColor\": \"Black\"\n              },\n              \"Sectors\": [\n                \"Pass\",\n                \"Fail\"\n              ]\n            }\n          ],\n          \"PieChart\": [\n            {\n              \"PieChartID\": 1,\n              \"PieChartValueID\": 0,\n              \"PlotEnable\": true,\n              \"PlotLabel\": \"Yeild Chart\",\n              \"PlotLabelFont\": {\n                \"FontName\": \"Times New Roman\",\n                \"FontSize\": 15,\n                \"IsBold\": true,\n                \"IsItalic\": false,\n                \"IsUnderline\": false,\n                \"IsStrikeout\": false,\n                \"FontColor\": \"Black\"\n              },\n              \"Sectors\": [\n                \"Pass\",\n                \"Fail\"\n              ]\n            }\n          ]\n        }\n      }\n    ]\n  },\n  \"UIParameters\": {\n    \"UIUpdateRate\": {\n      \"NumberOfImagesToBeDisplayed\": 1,\n      \"ImageCountWindow\": 5\n    },\n    \"ImageDisplay\": {\n      \"HorizontalCorrection\": 15,\n      \"VerticalCorrection\": 7,\n      \"ExtendedHeight\": 575,\n      \"SingleImageWidth\": 990,\n      \"SingleImageDisplay\": {\n        \"Width\": 480,\n        \"Height\": 273,\n        \"Top\": 29,\n        \"Left\": 0,\n        \"StringWidth\": 20,\n        \"StringHeight\": 24\n      },\n      \"MultipleImageDisplay\": [\n        {\n          \"Width\": 574,\n          \"Height\": 990,\n          \"Top\": 29,\n          \"Left\": 0,\n          \"StringWidth\": 20,\n          \"StringHeight\": 24\n        },\n        {\n          \"Width\": 20,\n          \"Height\": 20,\n          \"Top\": 29,\n          \"Left\": 0,\n          \"StringWidth\": 20,\n          \"StringHeight\": 24\n        },\n        {\n          \"Width\": 493,\n          \"Height\": 581,\n          \"Top\": 29,\n          \"Left\": 0,\n          \"StringWidth\": 20,\n          \"StringHeight\": 24\n        }\n      ]\n    },\n    \"CustomerLogoFilePath\": \"ZenGage v3.0 UI\\\\UX\\\\IMages\\\\fcilogo.png\",\n    \"ZentronLogoFilePath\": \"ZenGage v3.0 UI\\\\UX\\\\IMages\\\\ZenLogo(181x55).png\",\n    \"LoadingBarInitTime\": 6000,\n    \"DisplayCpCpkPopup\": true\n  }\n}"
  out "Data Out":T1
  out "Error Message":string
  in  "pathList":string[](array[string])=["$.Array[Name=1ABC2]"]
  out "VClusterOut":variant
  in  "error in":errorcluster
  in  "JSON String":path=path "E:/JSON File Handling/Path to VCluster/Data/Gtron System JSON 2nd June 2017.json"
  # "{\n\"History\": {\n    \"ZenParamsSpecVersion\": \"1.0.0\",\n    \"ModificationHistory\": [\n      {\n        \"DateModified\": \"19-07-2017\",\n        \"ModifiedBy\": \"SR\",\n        \"ModificationNotes\": \"FCI First version\",\n        \"DocumentVefrsion\": \"1.0.0\"\n      }\n    ],\n    \"ServiceHistory\": [\n      {\n        \"DateServiced\": \"23-03-2017\",\n        \"ServicedBy\": \"ABC\",\n        \"NextServiceDate\": \"23-03-2018\",\n        \"ServiceList\": {\n          \"CameraCalibrationDate\": \"2\",\n          \"CameraCalibrationFilePath\": \"C:\\\\Cam\",\n          \"SensorCalibration\": true,\n          \"SensorCalibNotes\": \"ReplacementDone\",\n          \"MotorCalib\": true,\n          \"MotorCalibNotes\": \"blah\"\n        },\n        \"ServiceNotes\": \"First version\"\n      },\n      {\n        \"DateServiced\": \"23-03-2017\",\n        \"ServicedBy\": \"ABC\",\n        \"NextServiceDate\": \"23-03-2018\",\n\"ServiceList\": {\n          \"CameraCalibrationDate\": \"2\",\n          \"CameraCalibrationFilePath\": \"C:\\\\Cam\",\n          \"SensorCalibration\": true,\n          \"SensorCalibNotes\": \"ReplacementDone\",\n          \"MotorCalib\": true,\n          \"MotorCalibNotes\": \"blah\"\n        },\n        \"ServiceNotes\": \"First version\"\n      }\n    ]\n  },\n  \"SystemParameters\": {\n    \"SystemName\": \"MolexGP2_001\",\n    \"SystemID\": \"GTRON1\",\n    \"CusftomerName\": \"Molex\",\n    \"Location\": \"Gandhinagar\",\n    \"InstallationfDate\": \"01-08-2015\",\n    \"NextServiceDate\": \"01-05-2017\",\n    \"CompatibleZenGageVersion\": \"2.0\",\n    \"NumberOfRacks\": 1,\n    \"TotalNumberOfCameras\": 3,\n    \"SoftwareFeatures\": {\n      \"ArduinoDiagnosticsEnableOnPowerOn\": true,\n      \"MotorDiagnosticsEnableOnPowerOn\": true,\n      \"CameraOpticsDiagnosticsEnableOnPowerOn\": false,\n      \"DefectTrackingEnable\": true,\n      \"AnalyticsEnable\": true,\n      \"DataLoggingEnable\": false,\n      \"ReportEnable\": false,\n      \"DeveloperMode\": false,\n      \"PauseOnReelCountFinish\": true,\n      \"PauseOnTotalCountFinish\": true,\n      \"DebugLevel\": 0,\n      \"SaveFailImages\": false\n    }\n  },\n  \"PartsConfigured\": [\n    {\n      \"Name\": \"102\",\n      \"NumberOfRack\": 1\n    }\n  ],\n  \"RackControllerParameters\": [\n    {\n      \"RackId\": 0,\n      \"PartsList\": [\n        {\n          \"Name\": \"102\",\n          \"ControlLimitsViolationThreshold\": {\n            \"M1\": 1,\n            \"N1\": 1\n          },\n          \"SpecificationLimitViolationThreshold\": {\n            \"M2\": 1,\n            \"N2\": 1\n          },\n          \"RejectPositionCount\": 106,\n          \"NumberOfCameras\": 1\n        },\n        {\n          \"Name\": \"122\",\n          \"ControlLimitsViolationThreshold\": {\n            \"M1\": 1,\n            \"N1\": 1\n          },\n          \"SpecificationLimitViolationThreshold\": {\n            \"M2\": 1,\n            \"N2\": 1\n          },\n          \"RejectPositionCount\": 77,\n          \"NumberOfCameras\": 3\n        },\n        {\n          \"Name\": \"145\",\n          \"ControlLimitsViolationThreshold\": {\n            \"M1\": 1,\n            \"N1\": 1\n          },\n          \"SpecificationLimitViolationThreshold\": {\n            \"M2\": 1,\n            \"N2\": 1\n          },\n          \"RejectPositionCount\": 78,\n          \"NumberOfCameras\": 3\n        },\n        {\n          \"Name\": \"162\",\n          \"ControlLimitsViolationThreshold\": {\n            \"M1\": 1,\n            \"N1\": 1\n          },\n          \"SpecificationLimitViolationThreshold\": {\n            \"M2\": 1,\n            \"N2\": 1\n          },\n          \"RejectPositionCount\": 78,\n          \"NumberOfCameras\": 3\n        },\n        {\n          \"Name\": \"182\",\n          \"ControlLimitsViolationThreshold\": {\n            \"M1\": 1,\n            \"N1\": 1\n          },\n          \"SpecificationLimitViolationThreshold\": {\n            \"M2\": 1,\n            \"N2\": 1\n          },\n          \"RejectPositionCount\": 78,\n          \"NumberOfCameras\": 3\n        },\n        {\n          \"Name\": \"175\",\n          \"ControlLimitsViolationThreshold\": {\n            \"M1\": 1,\n            \"N1\": 1\n          },\n          \"SpecificationLimitViolationThreshold\": {\n            \"M2\": 1,\n            \"N2\": 1\n          },\n          \"RejectPositionCount\": 78,\n          \"NumberOfCameras\": 3\n        },\n        {\n          \"Name\": \"130\",\n          \"ControlLimitsViolationThreshold\": {\n            \"M1\": 1,\n            \"N1\": 1\n          },\n          \"SpecificationLimitViolationThreshold\": {\n            \"M2\": 1,\n            \"N2\": 1\n          },\n          \"RejectPositionCount\": 78,\n          \"NumberOfCameras\": 3\n        },\n        {\n          \"Name\": \"142\",\n          \"ControlLimitsViolationThreshold\": {\n            \"M1\": 10,\n            \"N1\": 10\n          },\n          \"SpecificationLimitViolationThreshold\": {\n            \"M2\": 10,\n            \"N2\": 10\n          },\n          \"RejectPositionCount\": 78,\n          \"NumberOfCameras\": 3\n        },\n        {\n          \"Name\": \"160\",\n          \"ControlLimitsViolationThreshold\": {\n            \"M1\": 1,\n            \"N1\": 1\n          },\n          \"SpecificationLimitViolationThreshold\": {\n            \"M2\": 1,\n            \"N2\": 1\n          },\n          \"RejectPositionCount\": 78,\n          \"NumberOfCameras\": 3\n        }\n      ]\n    }\n  ],\n  \"CameraControllerParameters\": [\n    {\n      \"ID\": 0,\n      \"NoOfCameras\": 3,\n      \"CameraID\": [\n        0,\n        1,\n        2\n      ],\n      \"NoOfReceivers\": 1,\n      \"Diagnostics\": {\n        \"Path\": \"xxxxxx\",\n        \"LightCameraSequence\": [\n          {\n            \"Name\": \"LightCameraSequence1\",\n            \"CameraID\": 0,\n            \"LightID\": 1\n          },\n          {\n            \"Name\": \"LightCameraSequence2\",\n            \"CameraID\": 1,\n            \"LightID\": 2\n          },\n          {\n            \"Name\": \"LightCameraSequence3\",\n            \"CameraID\": 2,\n            \"LightID\": 3\n          }\n        ],\n        \"Delaytime\": 2000,\n        \"DecisionParameters\": {\n          \"Range\": [\n            70,\n            170\n          ],\n          \"AcceptancePercentage\": [\n            1,\n            20\n          ],\n          \"Comparison\": [\n            \"LesserThan\",\n            \"LesserThan\"\n          ],\n          \"AcceptableBlackBinValue\": 10000\n        },\n        \"DiagnosticsReceiverSequence\": {\n          \"ReceiverName\": \"RackController\",\n          \"ReceiverID\": 0\n        }\n      },\n      \"PartsList\": [\n        {\n          \"Name\": \"1891\",\n          \"CameraIDs\": [\n            0,\n            1\n          ],\n          \"ReceiverSequence\": [\n            {\n              \"ReceiverName\": \"Algorithm\",\n              \"ReceiverID\": 0,\n              \"NoOfActiveCameras\": 2\n            }\n          ]\n        },\n        {\n          \"Name\": \"1721\",\n          \"CameraIDs\": [\n            0,\n            1\n          ],\n          \"ReceiverSequence\": [\n            {\n              \"ReceiverName\": \"Algorithm\",\n              \"ReceiverID\": 0,\n              \"NoOfActiveCameras\": 2\n            }\n          ]\n        },\n        {\n          \"Name\": \"102\",\n          \"CameraIDs\": [\n            0\n          ],\n          \"ReceiverSequence\": [\n            {\n              \"ReceiverName\": \"RackController\",\n              \"ReceiverID\": 0,\n              \"NoOfActiveCameras\": 1\n            }\n          ]\n        },\n        {\n          \"Name\": \"122\",\n          \"CameraIDs\": [\n            0,\n            1,\n            2\n          ],\n          \"ReceiverSequence\": [\n            {\n              \"ReceiverName\": \"RackController\",\n              \"ReceiverID\": 0,\n              \"NoOfActiveCameras\": 3\n            }\n          ]\n        },\n        {\n          \"Name\": \"145\",\n          \"CameraIDs\": [\n            0,\n            1,\n            2\n          ],\n          \"ReceiverSequence\": [\n            {\n              \"ReceiverName\": \"RackController\",\n              \"ReceiverID\": 0,\n              \"NoOfActiveCameras\": 3\n            }\n          ]\n        },\n        {\n          \"Name\": \"162\",\n          \"CameraIDs\": [\n            0,\n            1,\n            2\n          ],\n          \"ReceiverSequence\": [\n            {\n              \"ReceiverName\": \"RackController\",\n              \"ReceiverID\": 0,\n              \"NoOfActiveCameras\": 3\n            }\n          ]\n        },\n        {\n          \"Name\": \"182\",\n          \"CameraIDs\": [\n            0,\n            1,\n            2\n          ],\n          \"ReceiverSequence\": [\n            {\n              \"ReceiverName\": \"RackController\",\n              \"ReceiverID\": 0,\n              \"NoOfActiveCameras\": 3\n            }\n          ]\n        },\n        {\n          \"Name\": \"175\",\n          \"CameraIDs\": [\n            0,\n            1,\n            2\n          ],\n          \"ReceiverSequence\": [\n            {\n              \"ReceiverName\": \"RackController\",\n              \"ReceiverID\": 0,\n              \"NoOfActiveCameras\": 3\n            }\n          ]\n        },\n        {\n          \"Name\": \"130\",\n          \"CameraIDs\": [\n            0,\n            1,\n            2\n          ],\n          \"ReceiverSequence\": [\n            {\n              \"ReceiverName\": \"RackController\",\n              \"ReceiverID\": 0,\n              \"NoOfActiveCameras\": 3\n            }\n          ]\n        },\n        {\n          \"Name\": \"142\",\n          \"CameraIDs\": [\n            0,\n            1,\n            2\n          ],\n          \"ReceiverSequence\": [\n            {\n              \"ReceiverName\": \"RackController\",\n              \"ReceiverID\": 0,\n              \"NoOfActiveCameras\": 3\n            }\n          ]\n        },\n        {\n          \"Name\": \"160\",\n          \"CameraIDs\": [\n            0,\n            1,\n            2\n          ],\n          \"ReceiverSequence\": [\n            {\n              \"ReceiverName\": \"RackController\",\n              \"ReceiverID\": 0,\n              \"NoOfActiveCameras\": 3\n            }\n          ]\n        }\n      ]\n    }\n  ],\n  \"ImageAcquisitionParameters\": [\n    {\n      \"Id\": 0,\n      \"SessionID\": \"Top Left\",\n      \"Type\": \"Top Left\",\n      \"Model\": \"Point grey CM3-U3-50S5m\",\n      \"InterfaceType\": \"USB3\",\n      \"SerialNumber\": \"x\",\n      \"Timeout\": 500,\n      \"GeneralCameraConfig\": [\n        {\n          \"ActiveAttribute\": \"TriggerMode\",\n          \"Value\": \"On\"\n        },\n        {\n          \"ActiveAttribute\": \"ExposureAuto\",\n          \"Value\": \"Off\"\n        },\n        {\n          \"ActiveAttribute\": \"ExposureTime\",\n          \"Value\": \"60\"\n        },\n        {\n          \"ActiveAttribute\": \"GainAuto\",\n          \"Value\": \"Off\"\n        },\n        {\n          \"ActiveAttribute\": \"Gain\",\n          \"Value\": \"0\"\n        }\n      ],\n      \"DefaultAOI\": [\n        1944,\n        1862,\n        474,\n        30\n      ],\n      \"DefaultReceiverSequence\": [\n        {\n          \"ReceiverID\": 0,\n          \"Index\": 0\n        }\n      ],\n      \"DefaultfileName\": \"ZenCAM\\\\Diagnostics\\\\Testimages\\\\top\",\n      \"Continuous\": 1,\n      \"NumberOfBuffers\": 150,\n      \"BufferNumberMode\": 0,\n      \"acquisitionTimeout\": 100,\n      \"ImageType\": 0,\n      \"Offline\": true,\n      \"ColorCameraParam\": {\n        \"PixelFormat\": \"BGRA 8 Packed\",\n        \"GammaEnable\": true,\n        \"GammaSelector\": \"sRGB\",\n        \"BalanceRationSelector\": [\n          \"Red\",\n          \"Blue\",\n          \"Green\"\n        ],\n        \"BalanceRationRaw\": [\n          95,\n          105,\n          115\n        ],\n        \"BalanceWhiteAuto\": \"Off\",\n        \"LightSourceSelector\": \"Daylight 5000 Kelvin\"\n      },\n      \"PartsList\": [\n        {\n          \"Name\": \"1891\",\n          \"ReceiverSequence\": [\n            {\n              \"ReceiverID\": 0,\n              \"Index\": 0\n            }\n          ],\n          \"AOI\": [\n            965,\n            650,\n            225,\n            250\n          ],\n          \"filePath\": \"ZenCam\\\\Test Images\\\\1891\\\\Rack1Top\"\n        },\n        {\n          \"Name\": \"1721\",\n          \"ReceiverSequence\": [\n            {\n              \"ReceiverID\": 0,\n              \"Index\": 0\n            }\n          ],\n          \"AOI\": [\n            1220,\n            670,\n            195,\n            200\n          ],\n          \"filePath\": \"ZenCam\\\\Test Images\\\\1721\\\\Rack1Top\"\n        },\n        {\n          \"Name\": \"102\",\n          \"ReceiverSequence\": [\n            {\n              \"ReceiverID\": 0,\n              \"Index\": 0\n            }\n          ],\n          \"AOI\": [\n            1600,\n            850,\n            300,\n            450\n          ],\n          \"filePath\": \"ZenCam\\\\Test Images\\\\102\\\\Top Left\"\n        },\n        {\n          \"Name\": \"122\",\n          \"ReceiverSequence\": [\n            {\n              \"ReceiverID\": 0,\n              \"Index\": 0\n            }\n          ],\n          \"AOI\": [\n            336,\n            1100,\n            1300,\n            278\n          ],\n          \"filePath\": \"ZenCam\\\\Test Images\\\\122\\\\Top Left\"\n        },\n        {\n          \"Name\": \"145\",\n          \"ReceiverSequence\": [\n            {\n              \"ReceiverID\": 0,\n              \"Index\": 0\n            }\n          ],\n          \"AOI\": [\n            480,\n            900,\n            1600,\n            500\n          ],\n          \"filePath\": \"ZenCam\\\\Test Images\\\\145\\\\Top Left\"\n        },\n        {\n          \"Name\": \"162\",\n          \"ReceiverSequence\": [\n            {\n              \"ReceiverID\": 0,\n              \"Index\": 0\n            }\n          ],\n          \"AOI\": [\n            400,\n            800,\n            1730,\n            440\n          ],\n          \"filePath\": \"ZenCam\\\\Test Images\\\\162\\\\Top Left\"\n        },\n        {\n          \"Name\": \"182\",\n          \"ReceiverSequence\": [\n            {\n              \"ReceiverID\": 0,\n              \"Index\": 0\n            }\n          ],\n          \"AOI\": [\n            464,\n            700,\n            1920,\n            600\n          ],\n          \"filePath\": \"ZenCam\\\\Test Images\\\\182\\\\Top Left\"\n        },\n        {\n          \"Name\": \"175\",\n          \"ReceiverSequence\": [\n            {\n              \"ReceiverID\": 0,\n              \"Index\": 0\n            }\n          ],\n          \"AOI\": [\n            448,\n            600,\n            2000,\n            850\n          ],\n          \"filePath\": \"ZenCam\\\\Test Images\\\\175\\\\Top Left\"\n        },\n        {\n          \"Name\": \"130\",\n          \"ReceiverSequence\": [\n            {\n              \"ReceiverID\": 0,\n              \"Index\": 0\n            }\n          ],\n          \"AOI\": [\n            400,\n            1000,\n            1420,\n            440\n          ],\n          \"filePath\": \"ZenCam\\\\Test Images\\\\130\\\\Top Left\"\n        },\n        {\n          \"Name\": \"142\",\n          \"ReceiverSequence\": [\n            {\n              \"ReceiverID\": 0,\n              \"Index\": 0\n            }\n          ],\n          \"AOI\": [\n            368,\n            930,\n            1550,\n            420\n          ],\n          \"filePath\": \"ZenCam\\\\Test Images\\\\142\\\\Top Left\"\n        },\n        {\n          \"Name\": \"160\",\n          \"ReceiverSequence\": [\n            {\n              \"ReceiverID\": 0,\n              \"Index\": 0\n            }\n          ],\n          \"AOI\": [\n            352,\n            940,\n            1800,\n            550\n          ],\n          \"filePath\": \"ZenCam\\\\Test Images\\\\160\\\\Top Left\"\n        }\n      ]\n    }\n  ],\n  \"AlgoParameters\": {\n    \"PartsList\": [\n      {\n        \"Name\": \"102\",\n        \"ImageStreams\": [\n          {\n            \"ThreadName\": \"TopRack\",\n            \"RackEnable\": true,\n            \"ThreadId\": 1,\n            \"RackId\": 1,\n            \"DifferenceParameter\": 1,\n            \"SplitCameraIDs\": [\n              0\n            ],\n            \"ImagingViews\": [\n              {\n                \"ViewName\": \"Top Left\",\n                \"ViewEnable\": true,\n                \"ImageID\": 1,\n                \"CameraID\": 0,\n                \"CalibrationFilePath\": \"Algorithm\\\\Calibration\\\\TL Calibrated Image\",\n                \"CalibImageFormat\": \"png\",\n                \"ReferenceCoordSystem\": {\n                  \"Method\": {\n                    \"Algo\": \"FCI Blob Circle\",\n                    \"BaseReference\": {\n                      \"OriginX\": 618,\n                      \"OriginY\": 464,\n                      \"Angle\": 178.38,\n                      \"AxisReference\": 0\n                    }\n                  },\n                  \"ROI\": [\n                    {\n                      \"ROI\": {\n                        \"Left\": 0,\n                        \"Top\": 260,\n                        \"Right\": 0,\n                        \"Bottom\": 700,\n                        \"Rotation\": 0\n                      },\n                      \"EdgeOptions\": {\n                        \"EdgePolarity\": 2,\n                        \"KernelSize\": 7,\n                        \"Width\": 5,\n                        \"MinimumEdgeStrength\": 50,\n                        \"InterpolationType\": 0,\n                        \"DataProcessingMethod\": 0\n                      },\n                      \"LineOptions\": {\n                        \"NumberofLines\": 1,\n                        \"Type\": 1,\n                        \"MinScore\": 10,\n                        \"MaxScore\": 1000,\n                        \"Orientation\": 0,\n                        \"AngleRange\": 30,\n                        \"AngleTolerance\": 10,\n                        \"StepSize\": 15,\n                        \"MinSNR\": 10,\n                        \"MinPoints\": 25,\n                        \"HoughIterations\": 5\n                      },\n                      \"Process\": 0,\n                      \"StepSize\": 10,\n                      \"SearchDirection\": 1,\n                      \"CircleEdgeOptions\": {\n                        \"SearchDirection\": 0,\n                        \"EdgeOptions\": {\n                          \"EdgePolarity\": 0,\n                          \"KernelSize\": 7,\n                          \"Width\": 5,\n                          \"MinimumEdgeStrength\": 50,\n                          \"InterpolationType\": 0,\n                          \"DataProcessingMethod\": 0\n                        }\n                      },\n                      \"CircleFitOptions\": {\n                        \"Process\": 3,\n                        \"StepSize\": 3,\n                        \"MAxPixelRadius\": 3\n                      },\n                      \"CircleSearchDirection\": 1,\n                      \"CurveParameters\": {\n                        \"ExtractionMode\": 0,\n                        \"EdgeThreshold\": 50,\n                        \"EdgeFilterSize\": 0,\n                        \"MinLength\": 25,\n                        \"RowSearchStepSize\": 15,\n                        \"ColSearchStepSize\": 15,\n                        \"MaxEndpointGap\": 10,\n                        \"Closed\": true,\n                        \"Subpixel\": true\n                      },\n                      \"MinimumMatchScore\": 800,\n                      \"CircleDescriptor\": {\n                        \"MinRadius\": 3,\n                        \"MaxRadius\": 200\n                      },\n                      \"EllipseDescriptor\": {\n                        \"MinMajorRadius\": 3,\n                        \"MaxMajorRadius\": 200,\n                        \"MinMinorRadius\": 3,\n                        \"MaxMinorRadius\": 100\n                      },\n                      \"ParallelLines\": {\n                        \"First\": 40,\n                        \"Second\": 55,\n                        \"Third\": 70\n                      }\n                    }\n                  ],\n                  \"Name\": \"FirstReference\",\n                  \"OverlayOptions\": {\n                    \"OverlayEnable\": false,\n                    \"OverlayText\": \"Height\",\n                    \"OverlayCoords\": [\n                      5,\n                      8\n                    ],\n                    \"OverlayAngle\": 56,\n                    \"OverlayTextSize\": 6,\n                    \"OverlayTextColor\": \"Blue\",\n                    \"OverlayROI\": true,\n                    \"OverlayRakeLine\": false,\n                    \"OverlayPoints\": false\n                  }\n                }\n              }\n            ]\n          }\n        ],\n        \"Measurements\": [\n          {\n            \"RackID\": 0,\n            \"ImageID\": 0,\n            \"CameraID\": 0,\n            \"MeasurementId\": 0,\n            \"Name\": \"EON Presence\",\n            \"AlgoName\": \"EON Presence 102\",\n            \"Type\": \"Max\",\n            \"MeasurementEnable\": true,\n            \"AlgorithmSequence\": {\n              \"RefernceEdge\": {\n                \"Enable\": true,\n                \"Method\": \"LineFinding\",\n                \"RefROI\": {\n                  \"Left\": 433,\n                  \"Top\": 292,\n                  \"Right\": 703,\n                  \"Bottom\": 665,\n                  \"Rotation\": 0\n                },\n                \"EdgeOptions\": {\n                  \"EdgePoarity\": 2,\n                  \"KernelSize\": 3,\n                  \"Width\": 3,\n                  \"MinimumEdgeStrength\": 50,\n                  \"InterpolationType\": 0,\n                  \"DataProcessingMethod\": 0\n                },\n                \"LineOptions\": {\n                  \"NumberofLines\": 1,\n                  \"Type\": 1,\n                  \"MinScore\": 10,\n                  \"MaxScore\": 1000,\n                  \"Orientation\": 0,\n                  \"AngleRange\": 10,\n                  \"AngleTolerance\": 1,\n                  \"StepSize\": 10,\n                  \"MinSNR\": 0,\n                  \"MinPoints\": 25,\n                  \"HoughIterations\": 5\n                },\n                \"SearchDirection\": 2\n              },\n              \"Measurement\": {\n                \"ROI1\": {\n                  \"Enable\": true,\n                  \"ROI\": {\n                    \"Left\": 0,\n                    \"Top\": 230,\n                    \"Right\": 0,\n                    \"Bottom\": 700,\n                    \"Rotation\": 0\n                  },\n                  \"EdgeOptions\": {\n                    \"EdgePoarity\": 0,\n                    \"KernelSize\": 3,\n                    \"Width\": 3,\n                    \"MinimumEdgeStrength\": 50,\n                    \"InterpolationType\": 0,\n                    \"DataProcessingMethod\": 0\n                  },\n                  \"LineOptions\": {\n                    \"NumberofLines\": 1,\n                    \"Type\": 1,\n                    \"MinScore\": 10,\n                    \"MaxScore\": 1000,\n                    \"Orientation\": 0,\n                    \"AngleRange\": 30,\n                    \"AngleTolerance\": 1,\n                    \"StepSize\": 3,\n                    \"MinSNR\": 0,\n                    \"MinPoints\": 25,\n                    \"HoughIterations\": 5\n                  },\n                  \"Process\": 1,\n                  \"StepSize\": 10,\n                  \"SearchDirection\": 0,\n                  \"CircleEdgeOptions\": {\n                    \"SearchDirection\": 0,\n                    \"EdgeOptions\": {\n                      \"EdgePoarity\": 2,\n                      \"KernelSize\": 3,\n                      \"Width\": 3,\n                      \"MinimumEdgeStrength\": 50,\n                      \"InterpolationType\": 1,\n                      \"DataProcessingMethod\": 1\n                    }\n                  },\n                  \"CircleFitOptions\": {\n                    \"Process\": 3,\n                    \"StepSize\": 3,\n                    \"MAxPixelRadius\": 3.85\n                  },\n                  \"CircleSearchDirection\": 1,\n                  \"CurveParameters\": {\n                    \"ExtractionMode\": 0,\n                    \"EdgeThreshold\": 50,\n                    \"EdgeFilterSize\": 0,\n                    \"MinLength\": 25,\n                    \"RowSearchStepSize\": 15,\n                    \"ColSearchStepSize\": 15,\n                    \"MaxEndpointGap\": 10,\n                    \"Closed\": true,\n                    \"Subpixel\": true\n                  },\n                  \"MinimumMatchScore\": 800,\n                  \"CircleDescriptor\": {\n                    \"MinRadius\": 3,\n                    \"MaxRadius\": 200\n                  },\n                  \"EllipseDescriptor\": {\n                    \"MinMajorRadius\": 2,\n                    \"MaxMajorRadius\": 200,\n                    \"MinMinorRadius\": 2,\n                    \"MaxMinorRadius\": 100\n                  }\n                },\n                \"ROI2\": {\n                  \"Enable\": true,\n                  \"ROI\": {\n                    \"Left\": 143,\n                    \"Top\": 244,\n                    \"Right\": 217,\n                    \"Bottom\": 456,\n                    \"Rotation\": 0.01\n                  },\n                  \"EdgeOptions\": {\n                    \"EdgePoarity\": 0,\n                    \"KernelSize\": 3,\n                    \"Width\": 3,\n                    \"MinimumEdgeStrength\": 50,\n                    \"InterpolationType\": 0,\n                    \"DataProcessingMethod\": 0\n                  },\n                  \"LineOptions\": {\n                    \"NumberofLines\": 1,\n                    \"Type\": 1,\n                    \"MinScore\": 10,\n                    \"MaxScore\": 1000,\n                    \"Orientation\": 0,\n                    \"AngleRange\": 30,\n                    \"AngleTolerance\": 1,\n                    \"StepSize\": 3,\n                    \"MinSNR\": 0,\n                    \"MinPoints\": 25,\n                    \"HoughIterations\": 5\n                  },\n                  \"Process\": 1,\n                  \"StepSize\": 10,\n                  \"SearchDirection\": 2,\n                  \"CircleEdgeOptions\": {\n                    \"SearchDirection\": 0,\n                    \"EdgeOptions\": {\n                      \"EdgePoarity\": 2,\n                      \"KernelSize\": 3,\n                      \"Width\": 3,\n                      \"MinimumEdgeStrength\": 50,\n                      \"InterpolationType\": 1,\n                      \"DataProcessingMethod\": 1\n                    }\n                  },\n                  \"CircleFitOptions\": {\n                    \"Process\": 3,\n                    \"StepSize\": 3,\n                    \"MAxPixelRadius\": 3.85\n                  },\n                  \"CircleSearchDirection\": 1,\n                  \"CurveParameters\": {\n                    \"ExtractionMode\": 0,\n                    \"EdgeThreshold\": 50,\n                    \"EdgeFilterSize\": 0,\n                    \"MinLength\": 25,\n                    \"RowSearchStepSize\": 15,\n                    \"ColSearchStepSize\": 15,\n                    \"MaxEndpointGap\": 10,\n                    \"Closed\": true,\n                    \"Subpixel\": true\n                  },\n                  \"MinimumMatchScore\": 800,\n                  \"CircleDescriptor\": {\n                    \"MinRadius\": 3,\n                    \"MaxRadius\": 200\n                  },\n                  \"EllipseDescriptor\": {\n                    \"MinMajorRadius\": 2,\n                    \"MaxMajorRadius\": 200,\n                    \"MinMinorRadius\": 2,\n                    \"MaxMinorRadius\": 100\n                  }\n                }\n              }\n            },\n            \"MathExpression\": {\n              \"Algorithm\": \"Default\",\n              \"MathExpression\": \"a = 1*a + 0\",\n              \"ResultVariable\": \"a\"\n            },\n            \"ResultVariableCluster\": {\n              \"RVName\": \"a\",\n              \"RVSequence\": \"MeasROI1\",\n              \"RVIndex\": 1,\n              \"RVID\": 1,\n              \"RVValue\": 22.6\n            },\n            \"CalibrationCoefficients\": {\n              \"A1\": 1,\n              \"A2\": 0,\n              \"A3\": 0\n            },\n            \"UserCalibCoefficients\": {\n              \"UserCorrectionLinearityCoeff\": 1,\n              \"UserCorrectionBiasCoeff\": 0\n            },\n            \"SpecValues\": {\n              \"LCL\": 1500,\n              \"UCL\": 2500,\n              \"LSL\": 1500,\n              \"USL\": 2500,\n              \"NominalValue\": 2000\n            },\n            \"OverlayOptions\": {\n              \"OverlayEnable\": false,\n              \"OverlayText\": \"Width\",\n              \"OverlayCoords\": [\n                5,\n                8\n              ],\n              \"OverlayAngle\": 56,\n              \"OverlayTextSize\": 6,\n              \"OverlayTextColor\": \"Blue\",\n              \"OverlayROI\": false,\n              \"OverlayRakeLine\": false,\n              \"OverlayPoints\": false\n            },\n            \"DatalogEnable\": true,\n            \"DisplayIcon\": \"C:\\\\Desktop\\\\displayimage.png\"\n          }\n        ]\n      }\n    ],\n    \"AlgoDefaultParameters\": {\n      \"AlgoName\": \"MaxClamp\",\n      \"Enable\": true,\n      \"AlgorithmSequenceDefault\": {\n        \"RefernceEdgeDefault\": {\n          \"Method\": \"LineFinding\",\n          \"RefROI\": {\n            \"Left\": 1014,\n            \"Top\": 95,\n            \"Right\": 1290,\n            \"Bottom\": 520,\n            \"Rotation\": 0\n          },\n          \"EdgeOptions\": {\n            \"EdgePoarity\": 0,\n            \"KernelSize\": 3,\n            \"Width\": 3,\n            \"MinimumEdgeStrength\": 50,\n            \"InterpolationType\": 1,\n            \"DataProcessingMethod\": 1\n          },\n          \"LineOptions\": {\n            \"NumberofLines\": 1,\n            \"Type\": 1,\n            \"MinScore\": 10,\n            \"MaxScore\": 1000,\n            \"Orientation\": 0,\n            \"AngleRange\": 10,\n            \"AngleTolerance\": 1,\n            \"StepSize\": 3,\n            \"MinSNR\": 0,\n            \"MinPoints\": 25,\n            \"HoughIterations\": 5\n          },\n          \"SearchDirection\": 2\n        },\n        \"MeasurementDefault\": {\n          \"ROI1\": {\n            \"ROI\": {\n              \"Left\": 100,\n              \"Top\": 150,\n              \"Right\": 400,\n              \"Bottom\": 700,\n              \"Rotation\": 0\n            },\n            \"EdgeOptions\": {\n              \"EdgePoarity\": 0,\n              \"KernelSize\": 3,\n              \"Width\": 3,\n              \"MinimumEdgeStrength\": 50,\n              \"InterpolationType\": 1,\n              \"DataProcessingMethod\": 1\n            },\n            \"LineOptions\": {\n              \"NumberofLines\": 1,\n              \"Type\": 1,\n              \"MinScore\": 10,\n              \"MaxScore\": 1000,\n              \"Orientation\": 0,\n              \"AngleRange\": 10,\n              \"AngleTolerance\": 1,\n              \"StepSize\": 3,\n              \"MinSNR\": 0,\n              \"MinPoints\": 25,\n              \"HoughIterations\": 5\n            },\n            \"Process\": 1,\n            \"StepSize\": 10,\n            \"SearchDirection\": 0,\n            \"CircleEdgeOptions\": {\n              \"SearchDirection\": 1,\n              \"EdgeOptions\": {\n                \"EdgePoarity\": 0,\n                \"KernelSize\": 3,\n                \"Width\": 3,\n                \"MinimumEdgeStrength\": 50,\n                \"InterpolationType\": 1,\n                \"DataProcessingMethod\": 1\n              }\n            },\n            \"CircleFitOptions\": {\n              \"Process\": 3,\n              \"StepSize\": 3,\n              \"MAxPixelRadius\": 3\n            },\n            \"CircleSearchDirection\": 1,\n            \"CurveParameters\": {\n              \"ExtractionMode\": 0,\n              \"EdgeThreshold\": 50,\n              \"EdgeFilterSize\": 0,\n              \"MinLength\": 25,\n              \"RowSearchStepSize\": 15,\n              \"ColSearchStepSize\": 15,\n              \"MaxEndpointGap\": 10,\n              \"Closed\": 0,\n              \"Subpixel\": 0\n            },\n            \"MinimumMatchScore\": 800,\n            \"CircleDescriptor\": {\n              \"MinRadius\": 3,\n              \"MaxRadius\": 200\n            },\n            \"EllipseDescriptor\": {\n              \"MinMajorRadius\": 2,\n              \"MaxMajorRadius\": 200,\n              \"MinMinorRadius\": 2,\n              \"MaxMinorRadius\": 100\n            },\n            \"OverlayOptions\": {\n              \"OverlayEnable\": true,\n              \"OverlayText\": \"Collar Width\",\n              \"OverlayCoords\": [\n                5,\n                8\n              ],\n              \"OverlayAngle\": 56,\n              \"OverlayTextSize\": 6,\n              \"OverlayTextColor\": \"Red\"\n            },\n            \"ResultVariable\": \"M1\"\n          },\n          \"ROI2\": {\n            \"ROI\": {\n              \"Left\": 100,\n              \"Top\": 150,\n              \"Right\": 400,\n              \"Bottom\": 700,\n              \"Rotation\": 0\n            },\n            \"EdgeOptions\": {\n              \"EdgePoarity\": 0,\n              \"KernelSize\": 3,\n              \"Width\": 3,\n              \"MinimumEdgeStrength\": 50,\n              \"InterpolationType\": 1,\n              \"DataProcessingMethod\": 1\n            },\n            \"LineOptions\": {\n              \"NumberofLines\": 1,\n              \"Type\": 1,\n              \"MinScore\": 10,\n              \"MaxScore\": 1000,\n              \"Orientation\": 0,\n              \"AngleRange\": 10,\n              \"AngleTolerance\": 1,\n              \"StepSize\": 3,\n              \"MinSNR\": 0,\n              \"MinPoints\": 25,\n              \"HoughIterations\": 5\n            },\n            \"Process\": 1,\n            \"StepSize\": 10,\n            \"SearchDirection\": 0,\n            \"CircleEdgeOptions\": {\n              \"SearchDirection\": 1,\n              \"EdgeOptions\": {\n                \"EdgePoarity\": 0,\n                \"KernelSize\": 3,\n                \"Width\": 3,\n                \"MinimumEdgeStrength\": 50,\n                \"InterpolationType\": 1,\n                \"DataProcessingMethod\": 1\n              }\n            },\n            \"CircleFitOptions\": {\n              \"Process\": 3,\n              \"StepSize\": 3,\n              \"MaxPixelRadius\": 3\n            },\n            \"CircleSearchDirection\": 1,\n            \"CurveParameters\": {\n              \"ExtractionMode\": 0,\n              \"EdgeThreshold\": 50,\n              \"EdgeFilterSize\": 0,\n              \"MinLength\": 25,\n              \"RowSearchStepSize\": 15,\n              \"ColSearchStepSize\": 15,\n              \"MaxEndpointGap\": 10,\n              \"Closed\": 0,\n              \"Subpixel\": 0\n            },\n            \"MinimumMatchScore\": 800,\n            \"CircleDescriptor\": {\n              \"MinRadius\": 3,\n              \"MaxRadius\": 200\n            },\n            \"EllipseDescriptor\": {\n              \"MinMajorRadius\": 2,\n              \"MaxMajorRadius\": 200,\n              \"MinMinorRadius\": 2,\n              \"MaxMinorRadius\": 100\n            },\n            \"OverlayOptions\": {\n              \"OverlayEnable\": true,\n              \"OverlayText\": \"Collar Width\",\n              \"OverlayCoords\": [\n                5,\n                8\n              ],\n              \"OverlayAngle\": 56,\n              \"OverlayTextSize\": 6,\n              \"OverlayTextColor\": \"Red\"\n            },\n            \"ResultVariable\": \"M2\"\n          }\n        },\n        \"MathExpressionDefault\": {\n          \"Algorithm\": \"Math1\",\n          \"MathExpression\": \"M2-M1\",\n          \"ResultVariable\": \"M3\"\n        }\n      },\n      \"CalibrationCoefficients\": {\n        \"A1\": 13,\n        \"A2\": 8.7,\n        \"A3\": 67.9\n      },\n      \"UserCalibCoefficients\": {\n        \"UserCorrectionBiasCoeff\": 56,\n        \"UserCorrectionLinearityCoeff\": 45\n      },\n      \"OverlayOptions\": {\n        \"OverlayEnable\": true,\n        \"OverlayText\": \"Collar Width\",\n        \"OverlayCoords\": [\n          5,\n          8\n        ],\n        \"OverlayAngle\": 56,\n        \"OverlayTextSize\": 6,\n        \"OverlayTextColor\": \"Red\"\n      },\n      \"DatalogEnable\": true,\n      \"DisplayIcon\": \"C:\\\\Desktop\\\\displayimage.png\"\n    }\n  },\n  \"MachineInterfaceRecipeOpcodes\": {\n    \"DeviceReadiness\": {\n      \"Ping\": [\n        \"01QRY1111\"\n      ],\n      \"PingResponse\": [\n        \"11YES11\"\n      ]\n    },\n    \"Initialization\": [\n      {\n        \"Clear\": [\n          \"01CLR1111\"\n        ]\n      },\n      {\n        \"Debug\": [\n          \"01DBG0011\"\n        ]\n      },\n      {\n        \"PinModeConfiguration\": [\n          \"01PMD39111\",\n          \"01PMD38111\",\n          \"01PMD40111\",\n          \"01PMD42111\",\n          \"01PMD16111\",\n          \"01PMD43111\",\n          \"01PMD34111\",\n          \"01PMD35111\",\n          \"01PMD36111\",\n          \"01PMD37111\",\n          \"01PMD30111\",\n          \"01PMD31111\",\n          \"01PMD32111\",\n          \"01PMD33111\",\n          \"01PMD46111\",\n          \"01PMD47111\",\n          \"01PMD48111\",\n          \"01PMD49111\",\n          \"01PMD13011\",\n          \"01PMD12011\",\n          \"01PMD11011\",\n          \"01PMD10011\",\n          \"01PMD09011\",\n          \"01PMD08011\",\n          \"01PMD02011\",\n          \"01PMD03011\",\n          \"01PMD05011\",\n          \"01PMD06011\",\n          \"01PMD04011\",\n          \"01PMD14011\",\n          \"01PMD52111\",\n          \"01PMD53111\",\n          \"01LOW3311\",\n          \"01LOW5211\",\n          \"01LOW5311\",\n          \"01HGH4211\",\n          \"01HGH1611\",\n          \"01HGH4311\",\n          \"01PMD07011\"\n        ]\n      },\n      {\n        \"EventSequenceOpcodes\": [\n          \"10ENT11341510430004100011\",\n          \"10ENT12361510410004150011\",\n          \"10ENT134211141029011\",\n          \"10ENT1439151523029011\",\n          \"10ENT15421210101011\",\n          \"10ENT161611171029011\",\n          \"10ENT1738151823029011\",\n          \"10ENT18161210101011\",\n          \"10ENT1943112101029011\",\n          \"10ENT210401521123029011\",\n          \"10ENT211431210101011\",\n          \"10ENT2124211213101511\",\n          \"10ENT213391521423025011\",\n          \"10ENT2144212215101011\",\n          \"10ENT2151611216101511\",\n          \"10ENT216381521723025011\",\n          \"10ENT2171612218101011\",\n          \"10ENT2184311219101511\",\n          \"10ENT219401522023025011\",\n          \"10ENT220431210101011\"\n        ]\n      },\n      {\n        \"LogicalOperations\": [\n          \"10LGC101010101011\"\n        ]\n      },\n      {\n        \"ConditionalOperations\": [\n          \"10CND10101011\"\n        ]\n      },\n      {\n        \"InterruptTriggerBindingOpcodes\": [\n          \"10SET2211111\",\n          \"10SET2221211\",\n          \"10SET2231311\",\n          \"10SET2241611\",\n          \"10SET2251911\",\n          \"10SET22621211\",\n          \"10SET2084100011\",\n          \"10SET2094100011\",\n          \"10SET2104100011\",\n          \"10SET2114100011\",\n          \"10SET2124100011\",\n          \"10SET2134100011\"\n        ]\n      },\n      {\n        \"PinInformation\": [\n          \"01STM4611\",\n          \"01WND4711\",\n          \"01S1U0411\",\n          \"01S1L0611\",\n          \"01S2U0511\",\n          \"01LOW3511\"\n        ]\n      }\n    ],\n    \"OpenLimitSwitchStatus\": [\n      {\n        \"LimitSwitchStatusCheck\": [\n          \"01PST0911\"\n        ],\n        \"LimitSwitchStatusResponse\": [\n          \"1109111\",\n          \"1109011\"\n        ]\n      }\n    ],\n    \"MotorDiagnostics\": [\n      {\n        \"GuideOpen\": [\n          \"01LOW3711\",\n          \"01ENL095500001111\",\n          \"10DLY55000011\",\n          \"01EVT2211\",\n          \"01LPI0911\"\n        ],\n        \"GuideOpenResponse\": [\n          \"11P0911\",\n          \"11W0911\"\n        ],\n        \"GuideClose\": [\n          \"01HGH3711\",\n          \"01ENL085500001111\",\n          \"10DLY55000011\",\n          \"01EVT2211\",\n          \"01LPI0811\"\n        ],\n        \"GuideCloseResponse\": [\n          \"11P0811\",\n          \"11W0811\"\n        ],\n        \"RotateReelerMotor\": [\n          \"10DLY4300011\",\n          \"01EVT2111\",\n          \"01LPI0011\"\n        ]\n      }\n    ],\n    \"HardwareButtonDiagnostics\": {\n      \"Run\": [\n        \"01ENL135500001111\",\n        \"01DBL1311\"\n      ],\n      \"Pause\": [\n        \"01ENL125500001111\",\n        \"01DBL1211\"\n      ],\n      \"Stop\": [\n        \"01ENL115500001111\",\n        \"01DBL1111\"\n      ],\n      \"BuzzerOff\": [\n        \"01ENL105500001111\",\n        \"01DBL1011\"\n      ]\n    },\n    \"TriggerLightCameraSequence\": [\n      {\n        \"Name\": \"LightCameraSequence1\",\n        \"On\": [\n          \"01EVT2311\"\n        ],\n        \"Off\": [\n          \"01HGH4211\"\n        ]\n      },\n      {\n        \"Name\": \"LightCameraSequence2\",\n        \"On\": [\n          \"01EVT2411\"\n        ],\n        \"Off\": [\n          \"01HGH1611\"\n        ]\n      },\n      {\n        \"Name\": \"LightCameraSequence3\",\n        \"On\": [\n          \"01EVT2511\"\n        ],\n        \"Off\": [\n          \"01HGH4311\"\n        ]\n      }\n    ],\n    \"SensorDiagnostics\": [\n      {\n        \"Name\": \"Sensor1\",\n        \"Opcodes\": [\n          \"01ENL025350001111\",\n          \"01SEN0211\",\n          \"01HGH4811\",\n          \"10SET20221211\"\n        ]\n      },\n      {\n        \"Name\": \"Sensor2\",\n        \"Opcodes\": [\n          \"01ENL035550001111\",\n          \"01SEN0311\",\n          \"01HGH4911\",\n          \"10SET20321211\"\n        ]\n      }\n    ],\n    \"TowerLampDiagnostics\": {\n      \"RedLamp\": [\n        \"01HGH3011\",\n        \"01LOW3011\"\n      ],\n      \"YellowLamp\": [\n        \"01HGH3111\",\n        \"01LOW3111\"\n      ],\n      \"GreenLamp\": [\n        \"01HGH3211\",\n        \"01LOW3211\"\n      ],\n      \"Buzzer\": [\n        \"01HGH3311\",\n        \"01LOW3311\"\n      ]\n    },\n    \"Select\": [\n      {\n        \"HardwareButtonStatus\": [\n          \"01ENL135550001111\",\n          \"01DBL1211\",\n          \"01DBL1111\",\n          \"01DBL1011\",\n          \"01DBL0811\",\n          \"01DBL0911\"\n        ]\n      },\n      {\n        \"SwitchOnYellow\": [\n          \"01HGH3111\"\n        ]\n      },\n      {\n        \"StampingWindingControl\": [\n          \"01LOW4611\",\n          \"01LOW4711\"\n        ]\n      }\n    ],\n    \"Run\": {\n      \"HardwareButtonStatus\": [\n        \"01LOW3511\",\n        \"01DBL1311\",\n        \"01ENL125500001111\",\n        \"01ENL115500001111\",\n        \"01DBL1011\",\n        \"01DBL0811\",\n        \"01DBL0911\",\n        \"01LOW4611\",\n        \"01LOW4711\"\n      ],\n      \"Pass\": {\n        \"TowerLampStatus\": [\n          \"01LOW3011\",\n          \"01LOW3111\",\n          \"01HGH3211\",\n          \"01LOW3311\"\n        ]\n      }\n    },\n    \"Pause\": {\n      \"PauseButtonPress\": [\n        {\n          \"StampingWindingControl\": [\n            \"01SMT2111\",\n            \"01HGH4611\",\n            \"01HGH4711\"\n          ]\n        },\n        {\n          \"StampingWindingControl\": [\n            \"01HGH4611\",\n            \"01HGH4711\"\n          ]\n        },\n        {\n          \"DisableSensor\": []\n        },\n        {\n          \"TowerLampStatus\": [\n            \"01LOW3011\",\n            \"01HGH3111\",\n            \"01LOW3211\",\n            \"01LOW3311\"\n          ]\n        },\n        {\n          \"HardwareButtonStatus\": [\n            \"01ENL135500001111\",\n            \"01DBL1211\",\n            \"01ENL115500001111\",\n            \"01DBL1011\",\n            \"01DBL0811\",\n            \"01DBL0911\"\n          ]\n        }\n      ],\n      \"Fail\": [\n        {\n          \"DisableSensors\": [\n            \"01SMT2111\"\n          ]\n        },\n        {\n          \"TowerLampStatus\": [\n            \"01HGH3011\",\n            \"01LOW3111\",\n            \"01LOW3211\",\n            \"01HGH3311\"\n          ]\n        },\n        {\n          \"HardwareButtonStatus\": [\n            \"01ENL135500001111\",\n            \"01DBL1211\",\n            \"01ENL115500001111\",\n            \"01ENL105500001111\",\n            \"01DBL0811\",\n            \"01DBL0911\"\n          ]\n        }\n      ],\n      \"BuzzerOffButtonPress\": [\n        \"01LOW3311\"\n      ]\n    },\n    \"Exit\": {\n      \"Shutdown\": [\n        \"01EXT1411\",\n        \"01ENL145500001111\",\n        \"01PWR5211\"\n      ]\n    },\n    \"DHBLS\": [\n      {\n        \"DisableHardwareButtons\": [\n          \"01DBL1311\",\n          \"01DBL1211\",\n          \"01DBL1111\",\n          \"01DBL1011\",\n          \"01DBL0811\",\n          \"01DBL0911\"\n        ]\n      },\n      {\n        \"TowerLampsOff\": [\n          \"01LOW3011\",\n          \"01LOW3111\",\n          \"01LOW3211\",\n          \"01LOW3311\"\n        ]\n      },\n      {\n        \"PowerOffSensors\": [\n          \"01LOW4811\",\n          \"01LOW4911\"\n        ]\n      },\n      {\n        \"DisableSensors\": [\n          \"01DBL0211\",\n          \"01DBL0311\"\n        ]\n      },\n      {\n        \"StampingWindingControl\": [\n          \"01HGH4611\",\n          \"01HGH4711\",\n          \"01SMT2111\"\n        ]\n      }\n    ],\n    \"PartsList\": [\n      {\n        \"Name\": \"102\",\n        \"RackDependentOpcodes\": [\n          {\n            \"MotorStepsForReadyToInsert\": [\n              \"01HGH3711\",\n              \"10DLY51350211\",\n              \"01EVT2211\",\n              \"01LPI0011\"\n            ],\n            \"MotorStepsForReadyToRun\": [\n              \"01HGH3711\",\n              \"10DLY4110311\",\n              \"01EVT2211\",\n              \"01LPI0011\"\n            ],\n            \"SetIndex\": [\n              \"10SET20220311\"\n            ],\n            \"EnableAndPowerOnSensor\": [\n              \"01ENL025350001111\",\n              \"01SEN0211\",\n              \"01HGH4811\",\n              \"01SST2111\"\n            ]\n          }\n        ]\n      },\n      {\n        \"Name\": \"182\",\n        \"RackDependentOpcodes\": [\n          {\n            \"MotorStepsForReadyToInsert\": [\n              \"01HGH3711\",\n              \"10DLY4367711\",\n              \"01EVT2211\",\n              \"01LPI0011\"\n            ],\n            \"MotorStepsForReadyToRun\": [\n              \"01HGH3711\",\n              \"10DLY4130311\",\n              \"01EVT2211\",\n              \"01LPI0011\"\n            ],\n            \"SetIndex\": [\n              \"10SET20221211\"\n            ],\n            \"EnableAndPowerOnSensor\": [\n              \"01ENL025350001111\",\n              \"01SEN0211\",\n              \"01HGH4811\",\n              \"01SST2111\"\n            ]\n          }\n        ]\n      },\n      {\n        \"Name\": \"145\",\n        \"RackDependentOpcodes\": [\n          {\n            \"MotorStepsForReadyToInsert\": [\n              \"01HGH3711\",\n              \"10DLY4521711\",\n              \"01EVT2211\",\n              \"01LPI0011\"\n            ],\n            \"MotorStepsForReadyToRun\": [\n              \"01HGH3711\",\n              \"10DLY4130311\",\n              \"01EVT2211\",\n              \"01LPI0011\"\n            ],\n            \"SetIndex\": [\n              \"10SET20221211\"\n            ],\n            \"EnableAndPowerOnSensor\": [\n              \"01ENL025350001111\",\n              \"01SEN0211\",\n              \"01HGH4811\",\n              \"01SST2111\"\n            ]\n          }\n        ]\n      },\n      {\n        \"Name\": \"142\",\n        \"RackDependentOpcodes\": [\n          {\n            \"MotorStepsForReadyToInsert\": [\n              \"01HGH3711\",\n              \"10DLY4890011\",\n              \"01EVT2211\",\n              \"01LPI0011\"\n            ],\n            \"MotorStepsForReadyToRun\": [\n              \"01HGH3711\",\n              \"10DLY395011\",\n              \"01EVT2211\",\n              \"01LPI0011\"\n            ],\n            \"SetIndex\": [\n              \"10SET20221211\"\n            ],\n            \"EnableAndPowerOnSensor\": [\n              \"01ENL025350001111\",\n              \"01SEN0211\",\n              \"01HGH4811\",\n              \"01SST2111\"\n            ]\n          }\n        ]\n      },\n      {\n        \"Name\": \"122\",\n        \"RackDependentOpcodes\": [\n          {\n            \"MotorStepsForReadyToInsert\": [\n              \"01HGH3711\",\n              \"10DLY51200411\",\n              \"01EVT2211\",\n              \"01LPI0011\"\n            ],\n            \"MotorStepsForReadyToRun\": [\n              \"01HGH3711\",\n              \"10DLY4110311\",\n              \"01EVT2211\",\n              \"01LPI0011\"\n            ],\n            \"SetIndex\": [\n              \"10SET20221211\"\n            ],\n            \"EnableAndPowerOnSensor\": [\n              \"01ENL025350001111\",\n              \"01SEN0211\",\n              \"01HGH4811\",\n              \"01SST2111\"\n            ]\n          }\n        ]\n      },\n      {\n        \"Name\": \"130\",\n        \"RackDependentOpcodes\": [\n          {\n            \"MotorStepsForReadyToInsert\": [\n              \"01HGH3711\",\n              \"10DLY4900011\",\n              \"01EVT2211\",\n              \"01LPI0011\"\n            ],\n            \"MotorStepsForReadyToRun\": [\n              \"01HGH3711\",\n              \"10DLY4110311\",\n              \"01EVT2211\",\n              \"01LPI0011\"\n            ],\n            \"SetIndex\": [\n              \"10SET20221211\"\n            ],\n            \"EnableAndPowerOnSensor\": [\n              \"01ENL025350001111\",\n              \"01SEN0211\",\n              \"01HGH4811\",\n              \"01SST2111\"\n            ]\n          }\n        ]\n      },\n      {\n        \"Name\": \"160\",\n        \"RackDependentOpcodes\": [\n          {\n            \"MotorStepsForReadyToInsert\": [\n              \"01HGH3711\",\n              \"10DLY4321111\",\n              \"01EVT2211\",\n              \"01LPI0011\"\n            ],\n            \"MotorStepsForReadyToRun\": [\n              \"01HGH3711\",\n              \"10DLY4110311\",\n              \"01EVT2211\",\n              \"01LPI0011\"\n            ],\n            \"SetIndex\": [\n              \"10SET20221211\"\n            ],\n            \"EnableAndPowerOnSensor\": [\n              \"01ENL025350001111\",\n              \"01SEN0211\",\n              \"01HGH4811\",\n              \"01SST2111\"\n            ]\n          }\n        ]\n      },\n      {\n        \"Name\": \"162\",\n        \"RackDependentOpcodes\": [\n          {\n            \"MotorStepsForReadyToInsert\": [\n              \"01HGH3711\",\n              \"10DLY4600011\",\n              \"01EVT2211\",\n              \"01LPI0011\"\n            ],\n            \"MotorStepsForReadyToRun\": [\n              \"01HGH3711\",\n              \"10DLY4110311\",\n              \"01EVT2211\",\n              \"01LPI0011\"\n            ],\n            \"SetIndex\": [\n              \"10SET20221211\"\n            ],\n            \"EnableAndPowerOnSensor\": [\n              \"01ENL025350001111\",\n              \"01SEN0211\",\n              \"01HGH4811\",\n              \"01SST2111\"\n            ]\n          }\n        ]\n      },\n      {\n        \"Name\": \"175\",\n        \"RackDependentOpcodes\": [\n          {\n            \"MotorStepsForReadyToInsert\": [\n              \"01HGH3711\",\n              \"10DLY1111\",\n              \"01EVT2211\",\n              \"01LPI0011\"\n            ],\n            \"MotorStepsForReadyToRun\": [\n              \"01HGH3711\",\n              \"10DLY4110311\",\n              \"01EVT2211\",\n              \"01LPI0011\"\n            ],\n            \"SetIndex\": [\n              \"10SET20221211\"\n            ],\n            \"EnableAndPowerOnSensor\": [\n              \"01ENL025350001111\",\n              \"01SEN0211\",\n              \"01HGH4811\",\n              \"01SST2111\"\n            ]\n          }\n        ]\n      }\n    ],\n    \"HardwareButtonPressed\": {\n      \"RunButtonPress\": [\n        \"11P1311\"\n      ],\n      \"PauseButtonPress\": [\n        \"11P1211\"\n      ],\n      \"StopButtonPress\": [\n        \"11P1111\"\n      ],\n      \"BuzzerOffButtonPress\": [\n        \"11P1011\"\n      ]\n    },\n    \"ReadyPositionReached\": [\n      \"11P0011\"\n    ],\n    \"IncorrectOpcode\": [\n      \"11FLS11\"\n    ]\n  },\n  \"AnalyticsParameters\": {\n    \"UpdateRateCategories\": {\n      \"LOW\": {\n        \"SampleElapsed\": 100,\n        \"TimeElapsed\": 4\n      },\n      \"MEDIUM\": {\n        \"SampleElapsed\": 20,\n        \"TimeElapsed\": 8\n      },\n      \"HIGH\": {\n        \"SampleElapsed\": 1,\n        \"TimeElapsed\": 5\n      }\n    },\n    \"AnalyticsForPartsList\": [\n      {\n        \"Name\": \"102\",\n        \"InitializationValues\": {\n          \"RowsIn2DArray\": 9000,\n          \"ColumnsIn2DArray\": 13,\n          \"SamplesToDisplay\": 100,\n          \"UpdateRate\": \"MEDIUM\"\n        },\n        \"PlotParameters\": {\n          \"Trend\": [\n            {\n              \"TrendID\": 1,\n              \"PlotEnable\": true,\n              \"PlotTitle\": \"EON Presence Summary\",\n              \"PlotCaptionFont\": {\n                \"FontName\": \"Times New Roman\",\n                \"FontSize\": 15,\n                \"IsBold\": true,\n                \"IsItalic\": false,\n                \"IsUnderline\": false,\n                \"IsStrikeout\": false,\n                \"FontColor\": \"Black\"\n              },\n              \"XLabel\": \"Frequency Count\",\n              \"XLabelFont\": {\n                \"FontName\": \"Times New Roman\",\n                \"FontSize\": 15,\n                \"IsBold\": true,\n                \"IsItalic\": false,\n                \"IsUnderline\": false,\n                \"IsStrikeout\": false,\n                \"FontColor\": \"Black\"\n              },\n              \"SamplesToDisplay\": 100,\n              \"Channels\": [\n                {\n                  \"Label\": \"EON Presence Value\",\n                  \"YLabelFont\": {\n                    \"FontName\": \"Times New Roman\",\n                    \"FontSize\": 15,\n                    \"IsBold\": true,\n                    \"IsItalic\": false,\n                    \"IsUnderline\": false,\n                    \"IsStrikeout\": false,\n                    \"FontColor\": \"Black\"\n                  },\n                  \"MeasurementID\": 1,\n                  \"PlotColor\": \"Pink\",\n                  \"PointShape\": \"circle\",\n                  \"ShowOnGraph\": true\n                }\n              ]\n            }\n          ],\n          \"Histogram\": [\n            {\n              \"HistogramID\": 1,\n              \"PlotEnable\": true,\n              \"PlotTitle\": \"EON Presence Histogram Summary\",\n              \"PlotLabelFont\": {\n                \"FontName\": \"Times New Roman\",\n                \"FontSize\": 15,\n                \"IsBold\": true,\n                \"IsItalic\": false,\n                \"IsUnderline\": false,\n                \"IsStrikeout\": false,\n                \"FontColor\": \"Black\"\n              },\n              \"XLabel\": \"Height count\",\n              \"XLabelFont\": {\n                \"FontName\": \"Calibri\",\n                \"FontSize\": 15,\n                \"IsBold\": true,\n                \"IsItalic\": false,\n                \"IsUnderline\": false,\n                \"IsStrikeout\": false,\n                \"FontColor\": \"Black\"\n              },\n              \"YLabel\": \"EON Presence Values\",\n              \"YLabelFont\": {\n                \"FontName\": \"Times New Roman\",\n                \"FontSize\": 15,\n                \"IsBold\": true,\n                \"IsItalic\": false,\n                \"IsUnderline\": false,\n                \"IsStrikeout\": false,\n                \"FontColor\": \"Black\"\n              },\n              \"MeasurementID\": 1,\n              \"PlotColor\": \"Pink\",\n              \"SamplesToDisplay\": 10\n            }\n          ],\n          \"BarPlot\": [\n            {\n              \"BarPlotID\": 1,\n              \"BarValuesID\": 0,\n              \"PlotEnable\": true,\n              \"PlotLabel\": \"Production Summary\",\n              \"PlotLabelFont\": {\n                \"FontName\": \"Times New Roman\",\n                \"FontSize\": 15,\n                \"IsBold\": true,\n                \"IsItalic\": false,\n                \"IsUnderline\": false,\n                \"IsStrikeout\": false,\n                \"FontColor\": \"Black\"\n              },\n              \"XLabel\": \" Terminal Production\",\n              \"XLabelFont\": {\n                \"FontName\": \"Times New Roman\",\n                \"FontSize\": 15,\n                \"IsBold\": true,\n                \"IsItalic\": false,\n                \"IsUnderline\": false,\n                \"IsStrikeout\": false,\n                \"FontColor\": \"Black\"\n              },\n              \"YLabel\": \"Total Production Count\",\n              \"YLabelFont\": {\n                \"FontName\": \"Times New Roman\",\n                \"FontSize\": 15,\n                \"IsBold\": true,\n                \"IsItalic\": false,\n                \"IsUnderline\": false,\n                \"IsStrikeout\": false,\n                \"FontColor\": \"Black\"\n              },\n              \"Sectors\": [\n                \"Pass\",\n                \"Fail\"\n              ]\n            }\n          ],\n          \"PieChart\": [\n            {\n              \"PieChartID\": 1,\n              \"PieChartValueID\": 0,\n              \"PlotEnable\": true,\n              \"PlotLabel\": \"Yeild Chart\",\n              \"PlotLabelFont\": {\n                \"FontName\": \"Times New Roman\",\n                \"FontSize\": 15,\n                \"IsBold\": true,\n                \"IsItalic\": false,\n                \"IsUnderline\": false,\n                \"IsStrikeout\": false,\n                \"FontColor\": \"Black\"\n              },\n              \"Sectors\": [\n                \"Pass\",\n                \"Fail\"\n              ]\n            }\n          ]\n        }\n      }\n    ]\n  },\n  \"UIParameters\": {\n    \"UIUpdateRate\": {\n      \"NumberOfImagesToBeDisplayed\": 1,\n      \"ImageCountWindow\": 5\n    },\n    \"ImageDisplay\": {\n      \"HorizontalCorrection\": 15,\n      \"VerticalCorrection\": 7,\n      \"ExtendedHeight\": 575,\n      \"SingleImageWidth\": 990,\n      \"SingleImageDisplay\": {\n        \"Width\": 480,\n        \"Height\": 273,\n        \"Top\": 29,\n        \"Left\": 0,\n        \"StringWidth\": 20,\n        \"StringHeight\": 24\n      },\n      \"MultipleImageDisplay\": [\n        {\n          \"Width\": 574,\n          \"Height\": 990,\n          \"Top\": 29,\n          \"Left\": 0,\n          \"StringWidth\": 20,\n          \"StringHeight\": 24\n        },\n        {\n          \"Width\": 20,\n          \"Height\": 20,\n          \"Top\": 29,\n          \"Left\": 0,\n          \"StringWidth\": 20,\n          \"StringHeight\": 24\n        },\n        {\n          \"Width\": 493,\n          \"Height\": 581,\n          \"Top\": 29,\n          \"Left\": 0,\n          \"StringWidth\": 20,\n          \"StringHeight\": 24\n        }\n      ]\n    },\n    \"CustomerLogoFilePath\": \"ZenGage v3.0 UI\\\\UX\\\\IMages\\\\fcilogo.png\",\n    \"ZentronLogoFilePath\": \"ZenGage v3.0 UI\\\\UX\\\\IMages\\\\ZenLogo(181x55).png\",\n    \"LoadingBarInitTime\": 6000,\n    \"DisplayCpCpkPopup\": true\n  }\n}"
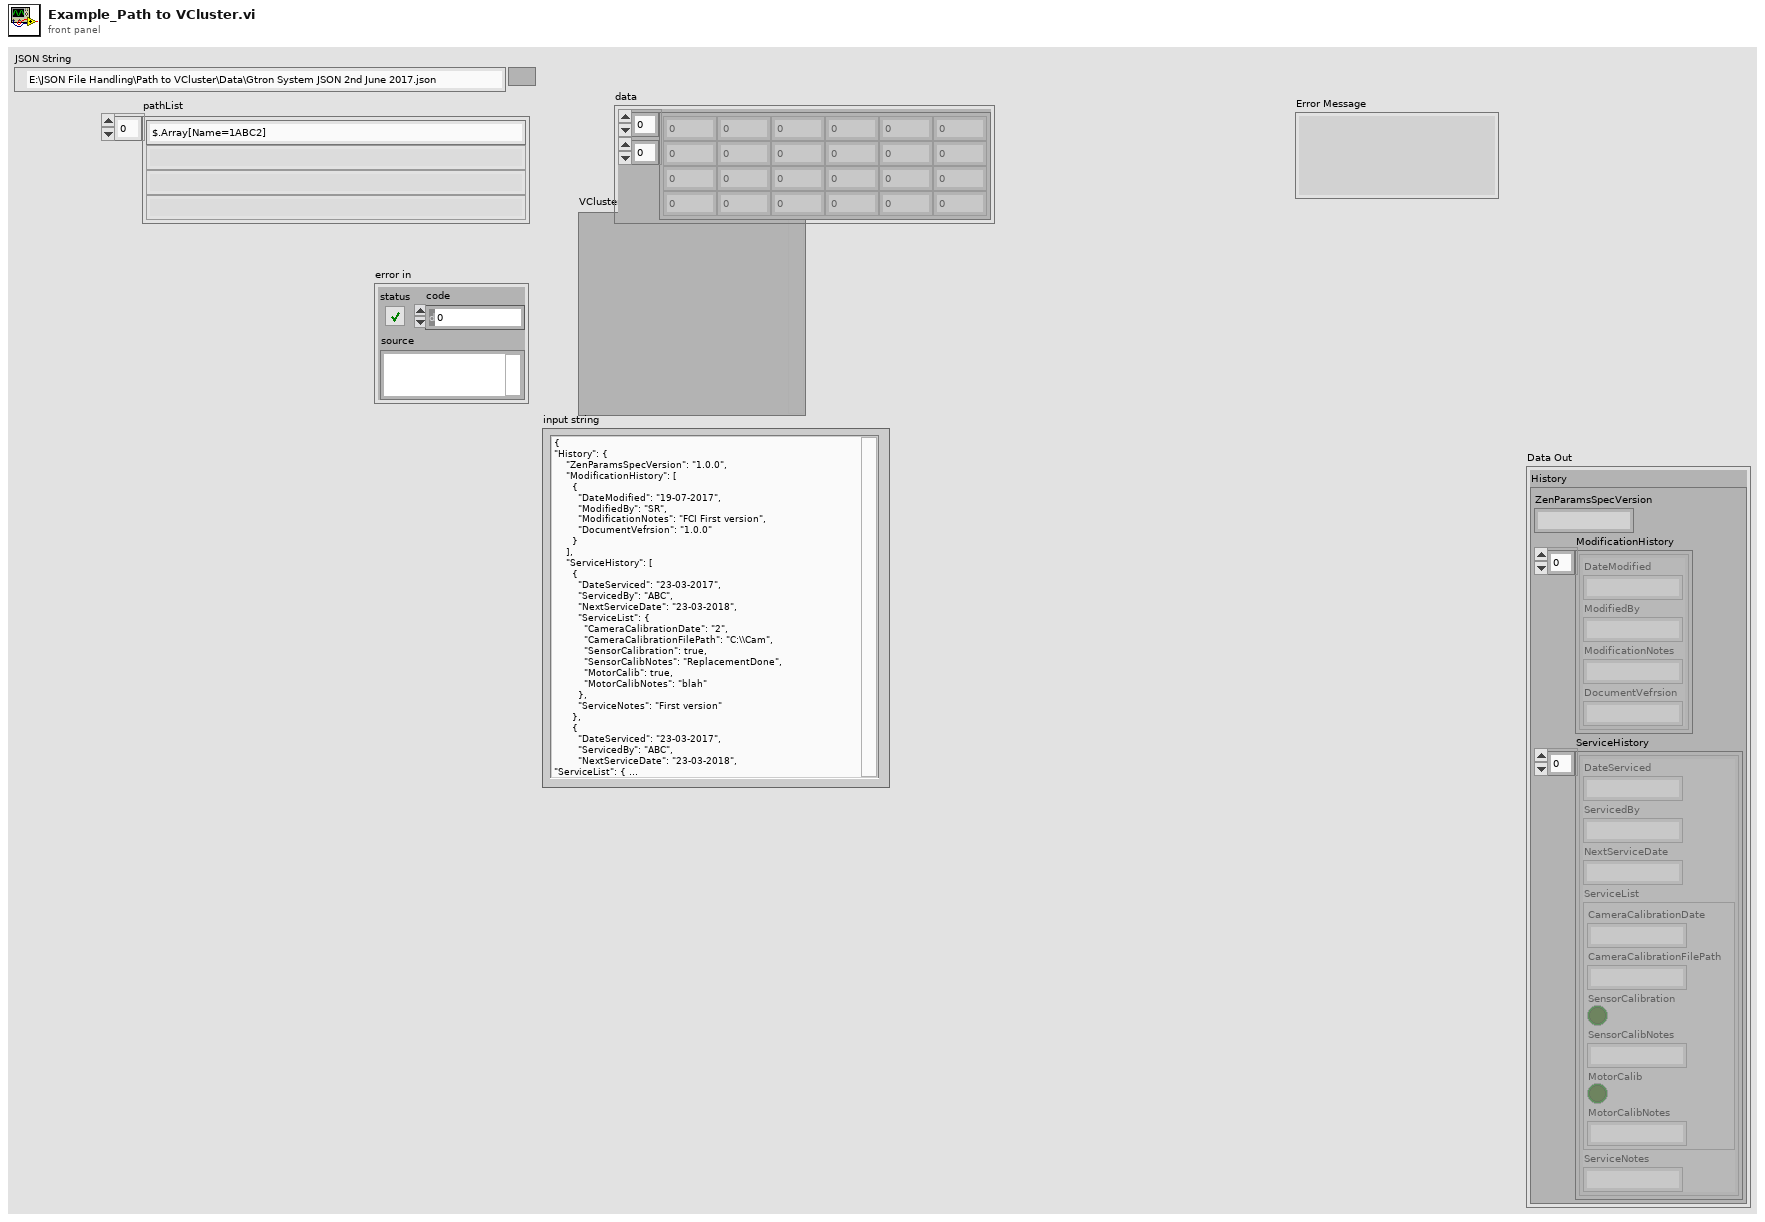
[diagram p1: front panel]
types:
  T1 = cluster{"History":cluster{"ZenParamsSpecVersion":string, "ModificationHistory":cluster{"DateModified":string, "ModifiedBy":string, "ModificationNotes":string, "DocumentVefrsion":string}[], "ServiceHistory":cluster{"DateServiced":string, "ServicedBy":string, "NextServiceDate":string, "ServiceList":cluster{"CameraCalibrationDate":string, "CameraCalibrationFilePath":string, "SensorCalibration":bool, "SensorCalibNotes":string, "MotorCalib":bool, "MotorCalibNotes":string}, "ServiceNotes":string}[]}}
  T2 = enum16{"open", "replace", "create", "open or create", "replace or create", "replace or create with confirmation"}
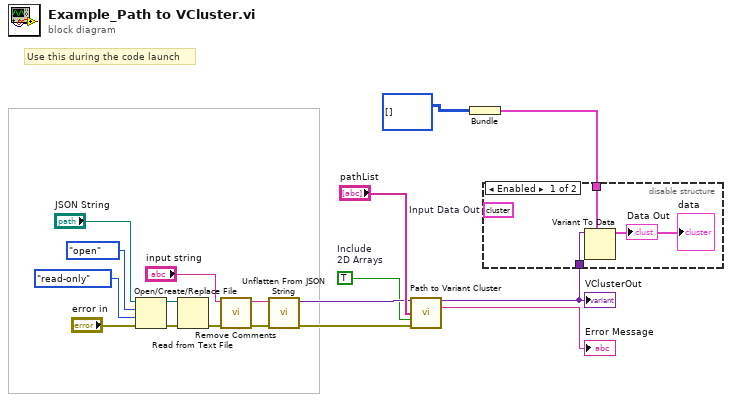
[diagram p0: block diagram]
diagram:
  w6 = TRUE  # Include 2D Arrays
  # "Use this during the code launch"
  n1 = Open/Create/Replace File(file path (use dialog)="JSON String", error in="error in", operation (0:open)=T2."open", access (0:read/write)=enum16{"read/write", "read-only", "write-only"}."read-only") -> (refnum out=w18:refnum<file>, error out=w4:errorcluster)  [unwired: 2 in, 1 out]
  n2 = Read from Text File(file (use dialog)=w18, error in=w4) -> (error out=w10:errorcluster)  [unwired: 2 in, 3 out]
  n3 = call "Remove Comments.vi"("error in (no error)"=w10, "input string"="input string") -> ("error out"=w12:errorcluster, "output String"=w8:string)  [unwired: 8 in]
  n4 = call <vilib>:"Unflatten From JSON String.vi"("error in (no error)"=w12, "JSON String"=w8) -> ("error out"=w11:errorcluster, "Variant"=w7:variant)  [unwired: 8 in]
  n5 = call "Path to Variant Cluster.vi"("VCluster in"=w7, "pathList"="pathList", "Include\n2D Arrays"=w6, "error IO"=w11) -> ("VCluster\n out"=w3:variant, "Error Message"=→"Error Message":string)  [unwired: 9 in, 1 out]
  "VClusterOut" <- w3
  n6 = Bundle(i32[][] []) -> (w1:cluster{i32[][]})  [unwired: 1 in]
  n7 = disable-structure shown="Enabled" {
    disable-tunnel: w3 -> [w21 _]
    disable-tunnel: w1 -> [w20 _]
    frame Enabled {
      (unwired) T1 {"History"={"ZenParamsSpecVersion"="1.0.0", "ModificationHistory"=[{"DateModified"="19-07-2017", "ModifiedBy"="SR", "ModificationNotes"="FCI First version", "DocumentVefrsion"="1.0.0"}], "ServiceHistory"=[{"DateServiced"="23-03-2017", "ServicedBy"="ABC", "NextServiceDate"="23-03-2018", "ServiceList"={"CameraCalibrationDate"="2", "CameraCalibrationFilePath"="C:\\Cam", "SensorCalibration"=TRUE, "SensorCalibNotes"="ReplacementDone", "MotorCalib"=TRUE, "MotorCalibNotes"="blah"}, "ServiceNotes"="First version"}, {"DateServiced"="23-03-2017", "ServicedBy"="ABC", "NextServiceDate"="23-03-2018", "ServiceList"={"CameraCalibrationDate"="2", "CameraCalibrationFilePath"="C:\\Cam", "SensorCalibration"=TRUE, "SensorCalibNotes"="ReplacementDone", "MotorCalib"=TRUE, "MotorCalibNotes"="blah"}, "ServiceNotes"="First version"}]}}  # Input Data Out
      n8 = Variant To Data(type=w20, Variant=w21) -> (data=→"data":cluster{i32[][]})  [unwired: 1 in, 1 out]
    }
    frame Disabled {
    }
  }
